vi "Modbus Message Loop.vi"(0 "Message Queues in":T1, 1 "PLC IP address":string="10.2.0.11", 3 "error in (no error)":errorcluster) -> (10 "error out":errorcluster)   [LabVIEW 2020, in "Modbus.lvlib"]
uses:
  Modbus.lvlib
  support/Message Queue/All Message Queues.ctl
  support/Message Queue/Message Cluster.ctl
  <vilib>/NI/Modbus Library/API/Master/Modbus Master.lvclass
  support/Message Queue/Enqueue Message (Single).vi
  <vilib>/NI/Modbus Library/API/Wrapper/Create TCP Master.vi
  support/Message Queue/Message Queue.lvlib
  <vilib>/NI/Modbus Library/API/Wrapper/API Main.lvlib
panel:
  out "appended array":string[](array[string])
  out "TimeoutRequestGetDataLDO":u16[](array[numeric])
  out "LDO Number":u32
  out "LDO Output":bool[](array[boolean])
  out "FV Number":u32
  out "Loop Count":i32
  out "FV Output":bool[](array[boolean])
  out "TimeoutRequestGetDataFVIR":i32[](array[numeric])
  out "Input Registers":u16[](array[numeric])
  # "Anybus: 192.168.0.50\nPLC: 192.168.0.20\n\nThis is available in the front HMI, e. IP and port. Useful for debugging and IP config change"
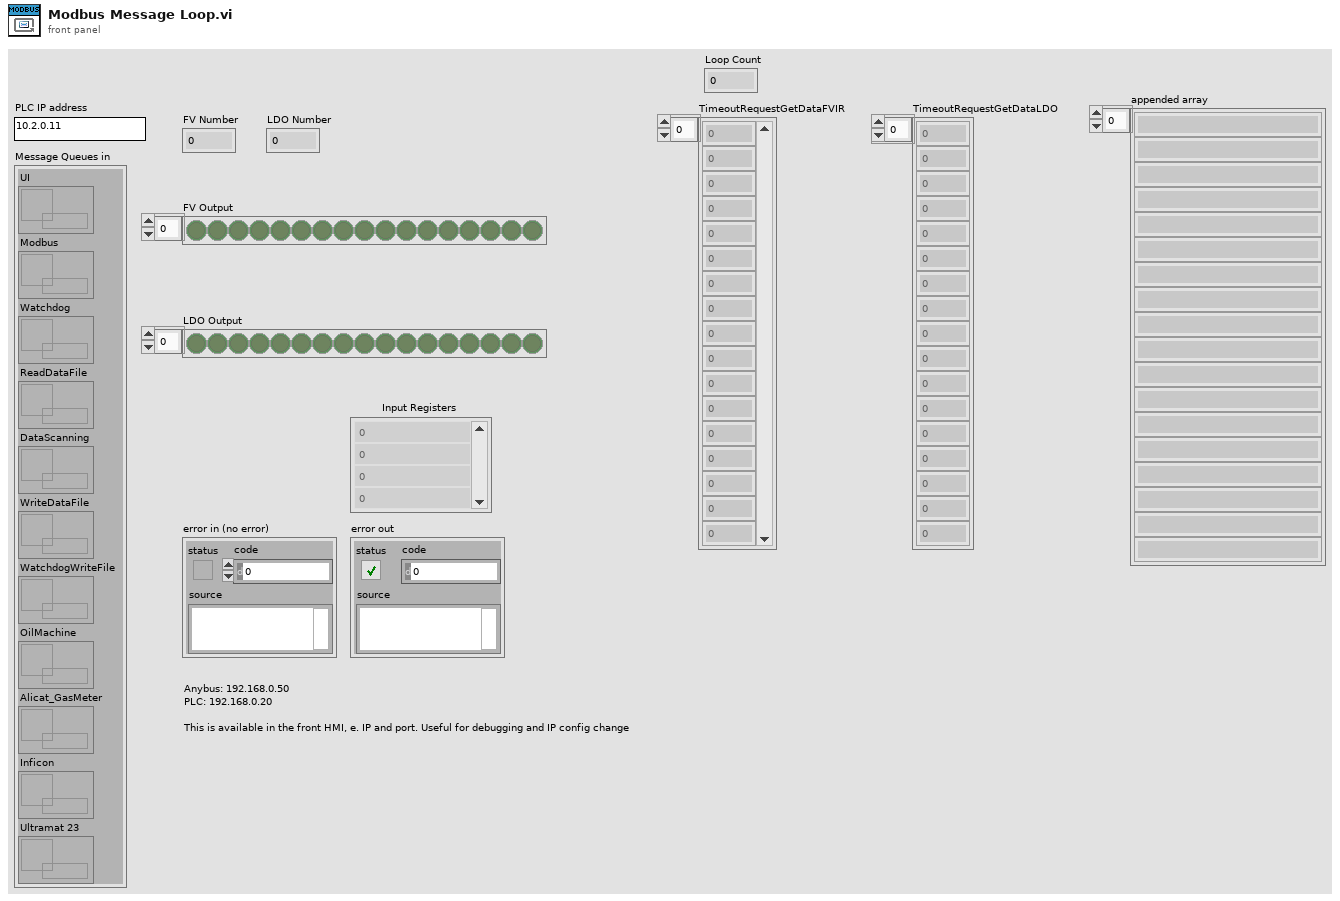
[diagram p1: front panel]
types:
  T1 = typedef "Message Queue.lvlib/All Message Queues.ctl" = cluster{"UI":refnum<queue>, "Modbus":refnum<queue>, "Watchdog":refnum<queue>, "ReadDataFile":refnum<queue>, "DataScanning":refnum<queue>, "WriteDataFile":refnum<queue>, "WatchdogWriteFile":refnum<queue>, "OilMachine":refnum<queue>, "Alicat_GasMeter":refnum<queue>, "Inficon":refnum<queue>, "Ultramat 23":refnum<queue>}
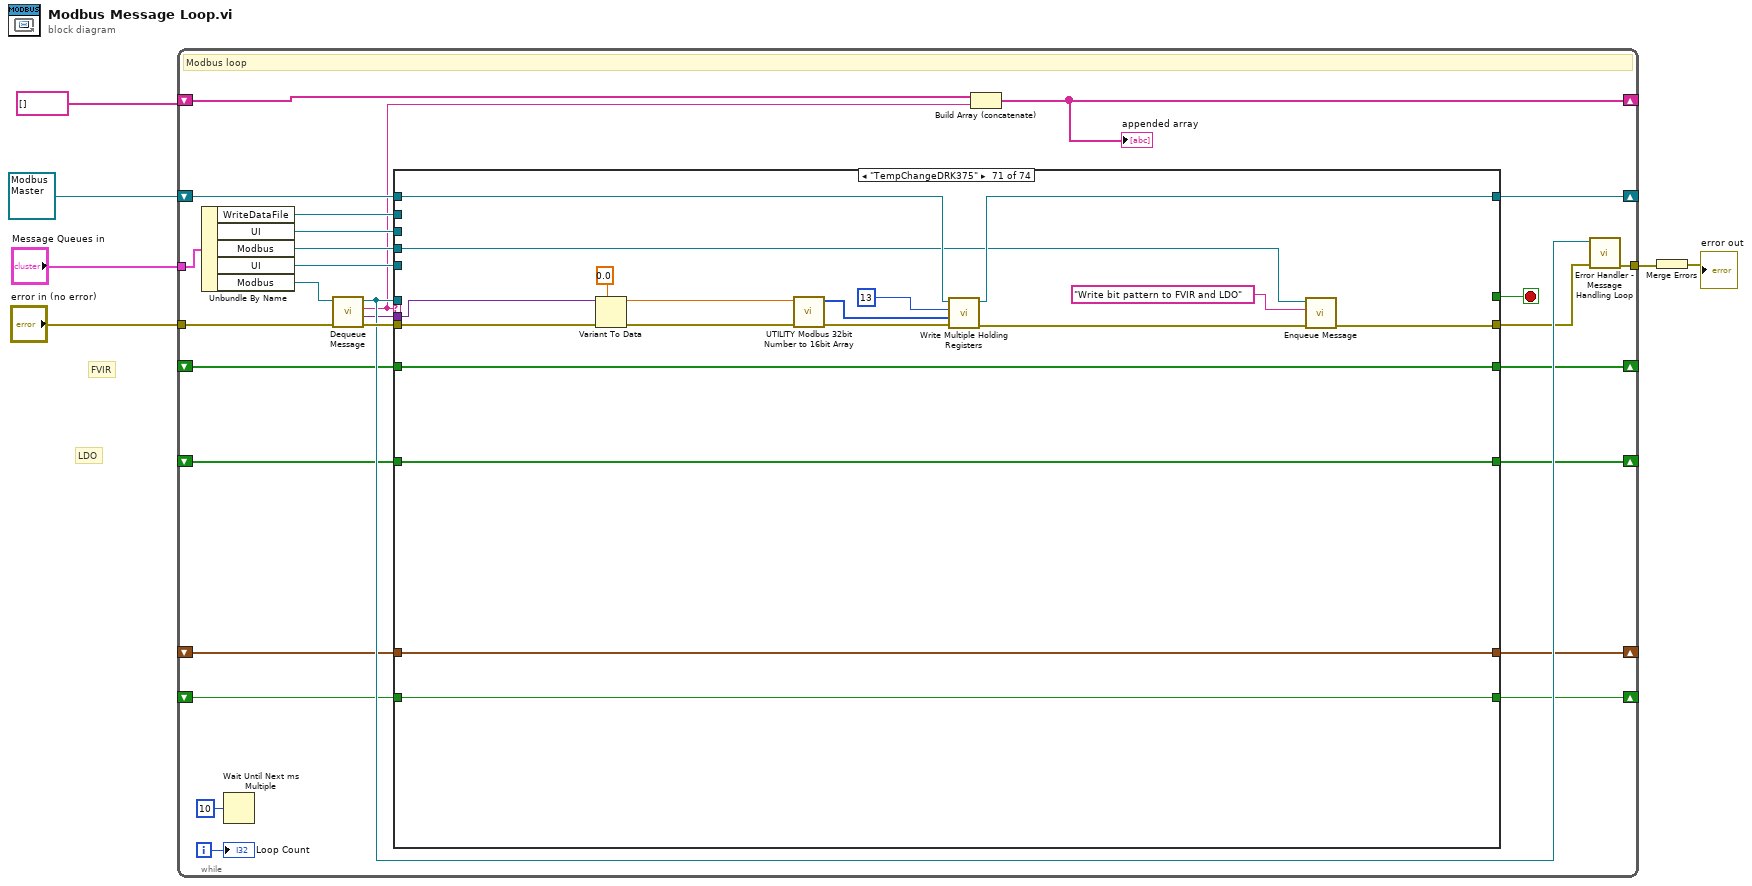
[diagram p0: block diagram]
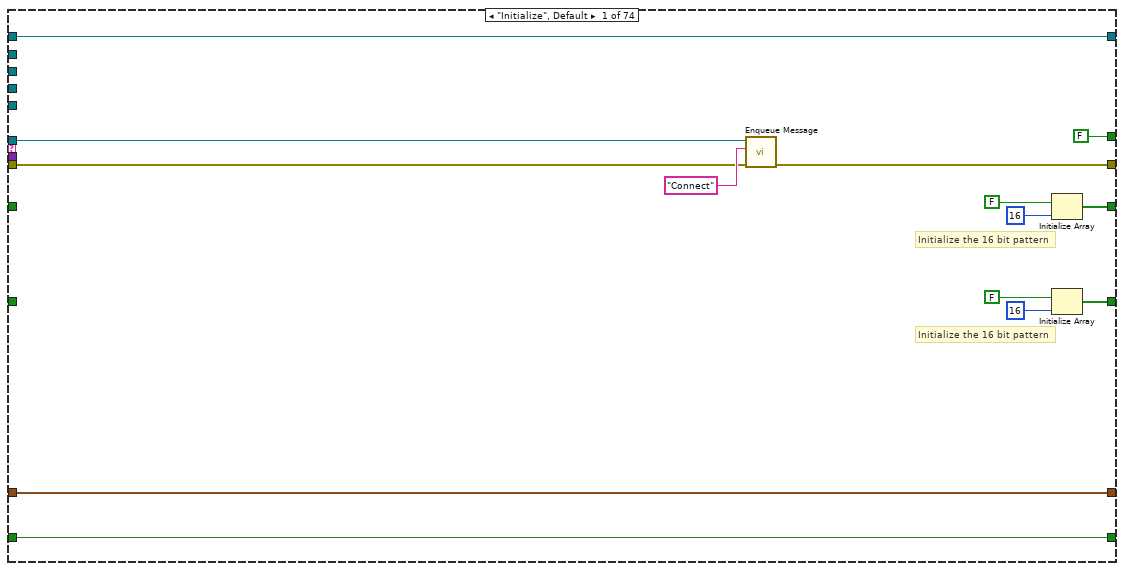
[diagram p2: hidden frame]
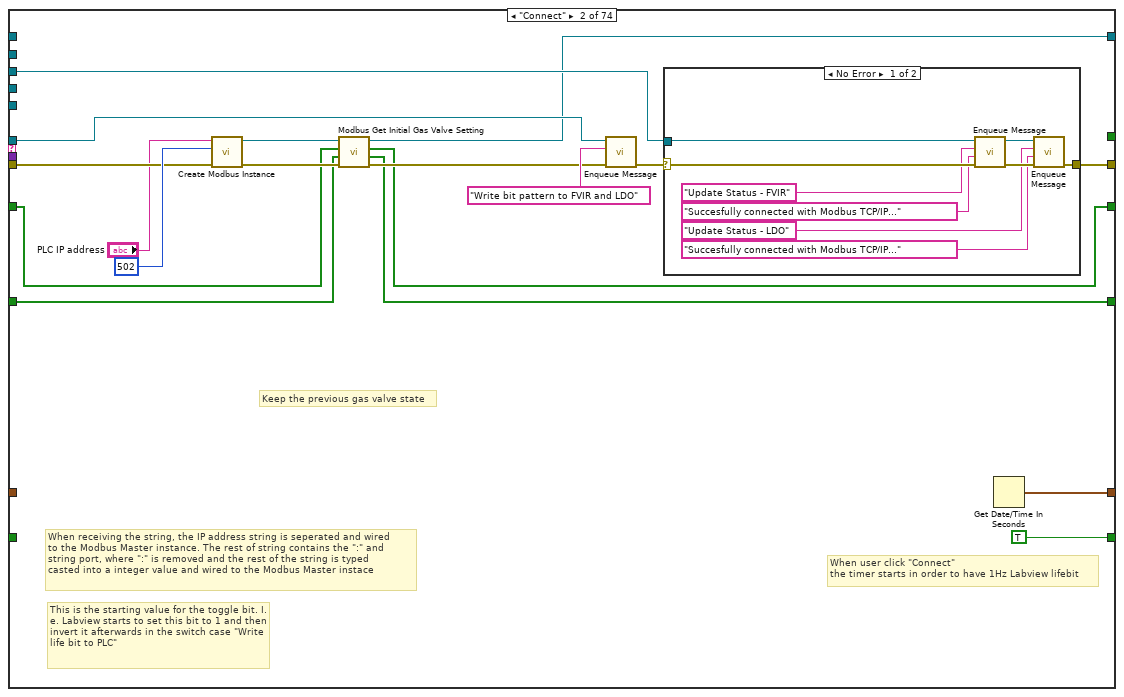
[diagram p3: hidden frame]
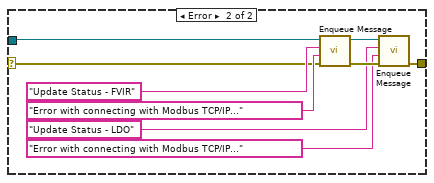
[diagram p4: hidden frame]
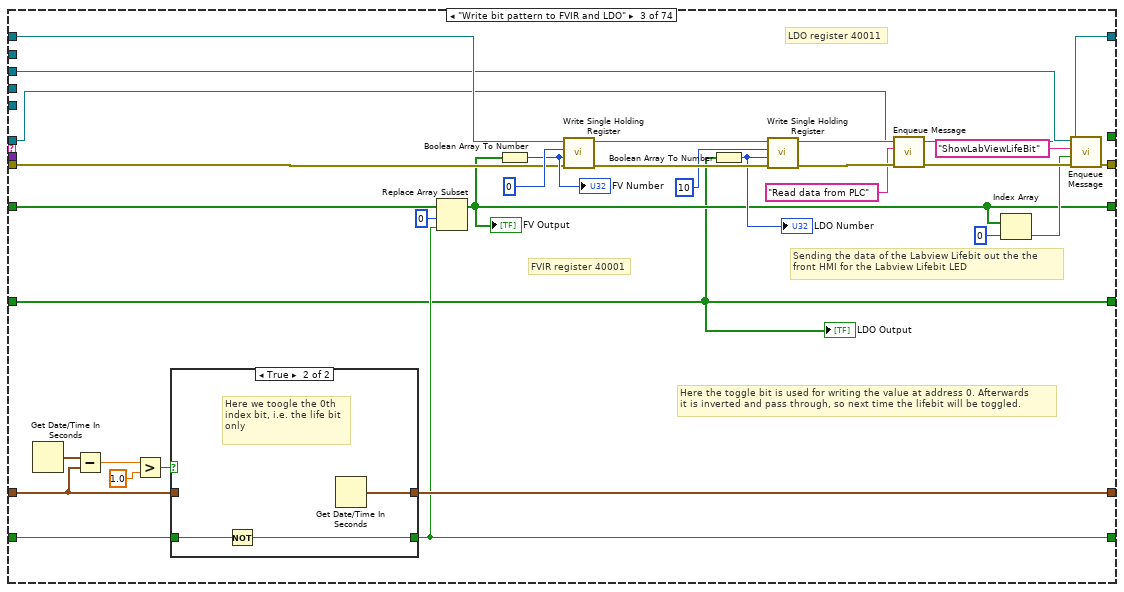
[diagram p5: hidden frame]
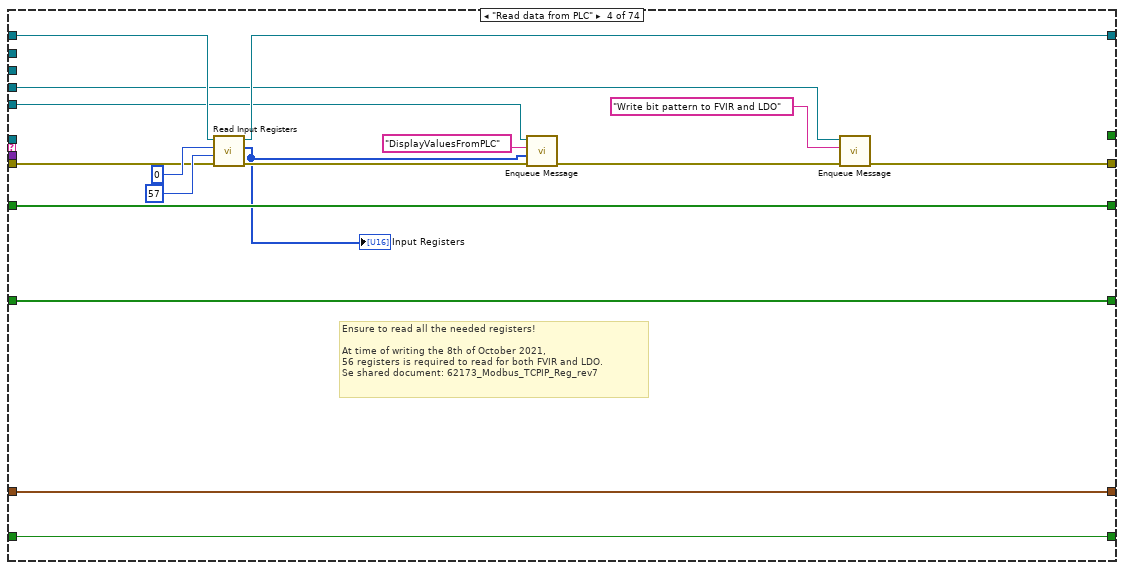
[diagram p7: hidden frame]
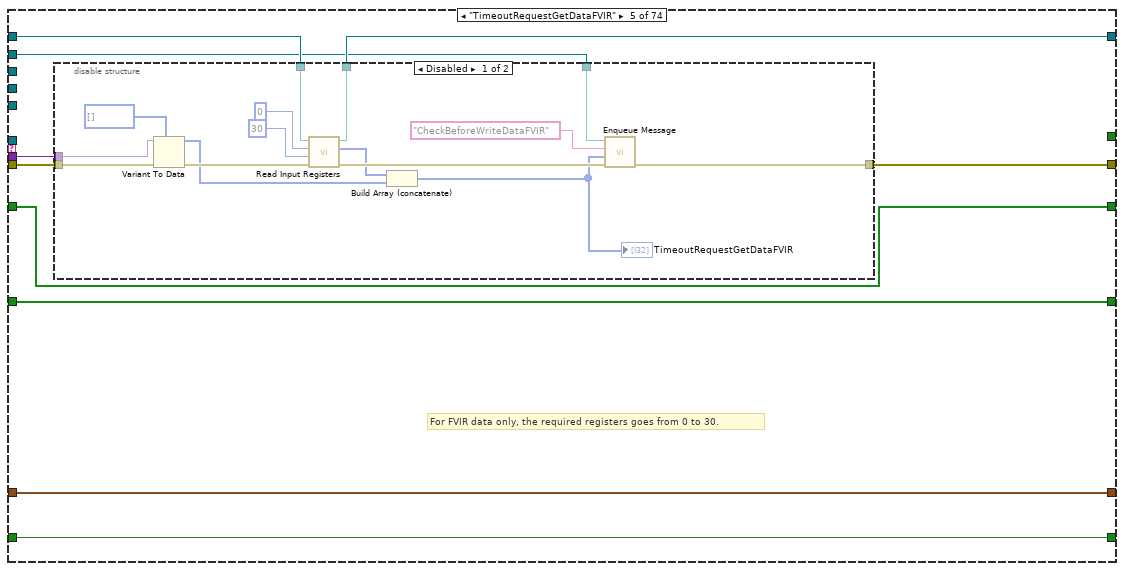
[diagram p8: hidden frame]
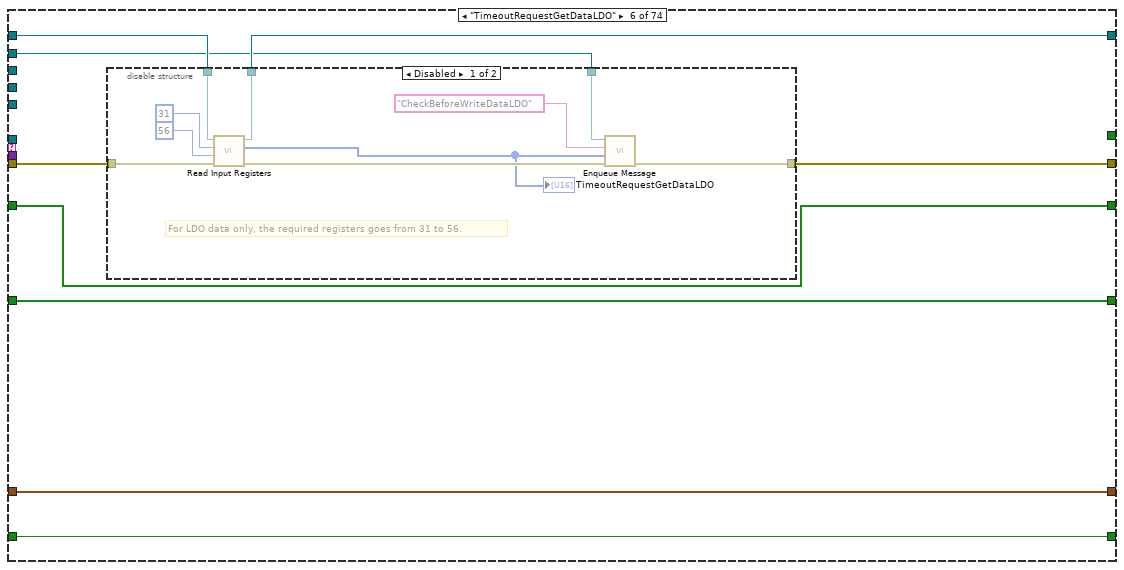
[diagram p10: hidden frame]
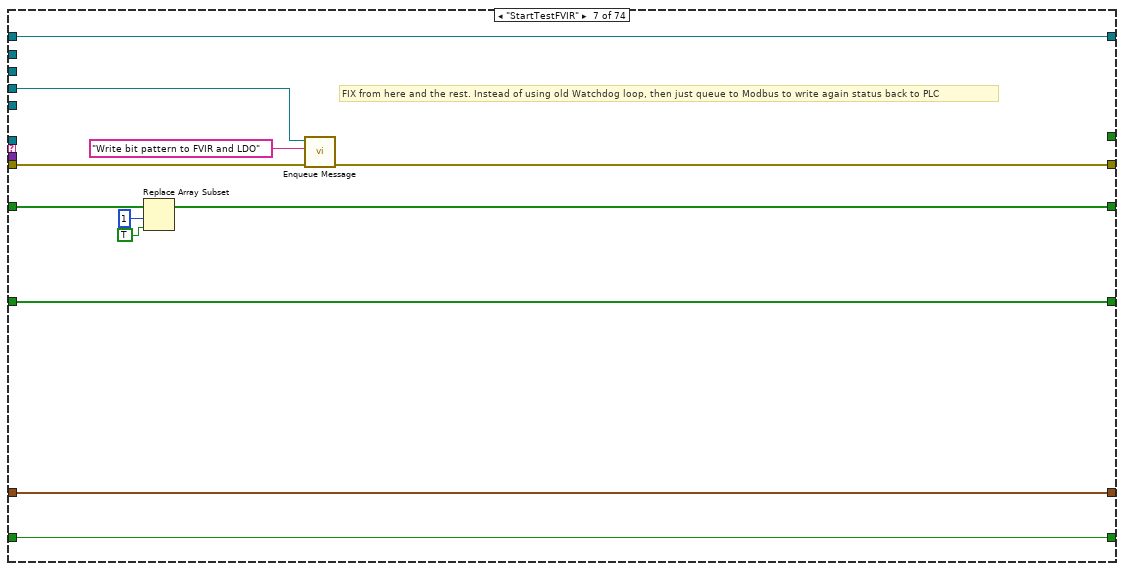
[diagram p12: hidden frame]
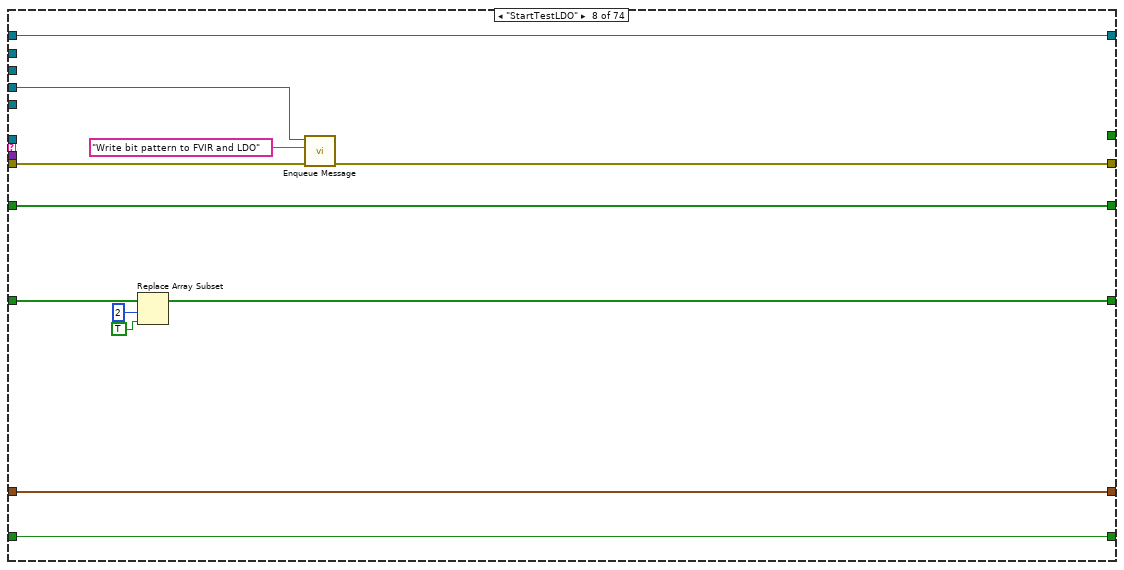
[diagram p13: hidden frame]
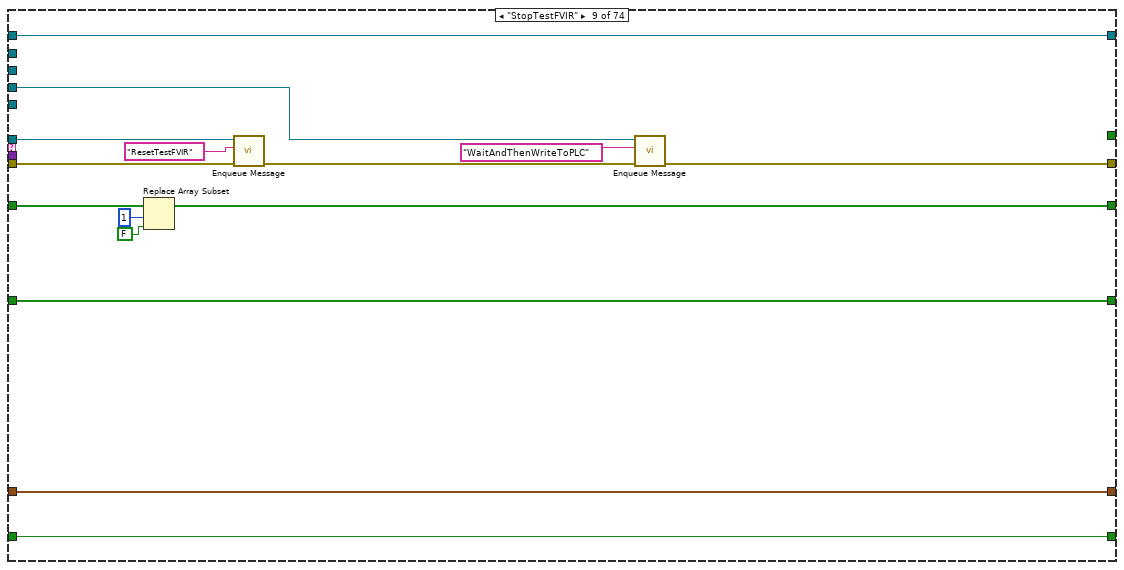
[diagram p14: hidden frame]
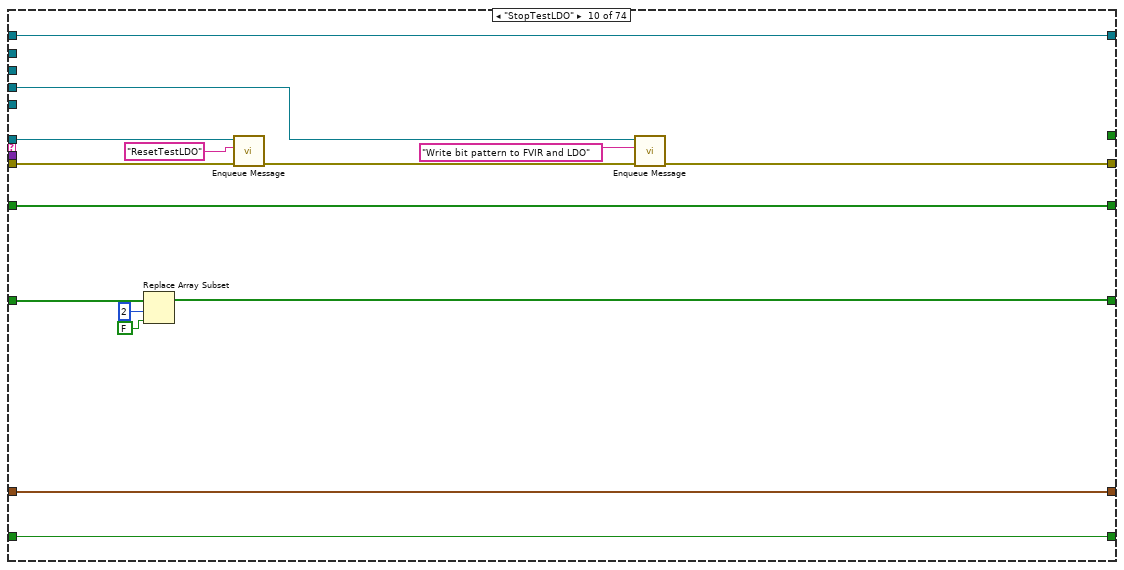
[diagram p15: hidden frame]
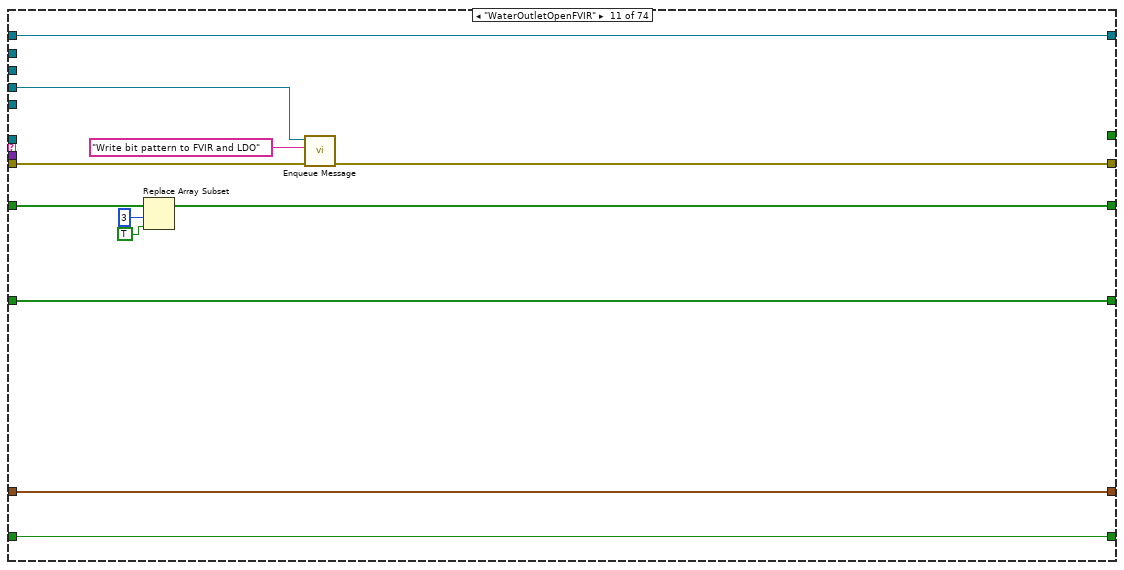
[diagram p16: hidden frame]
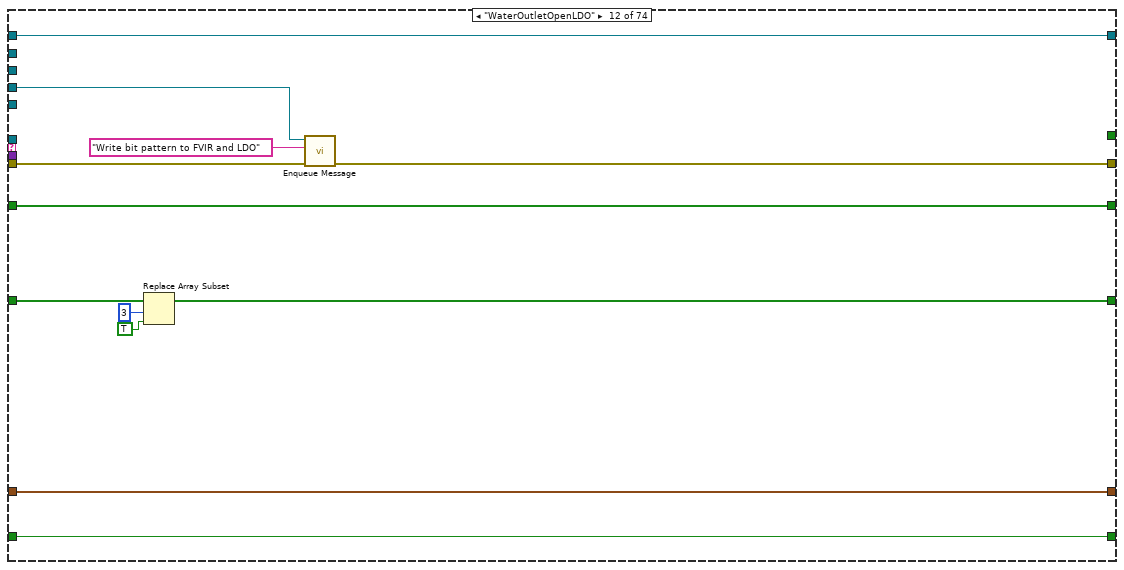
[diagram p17: hidden frame]
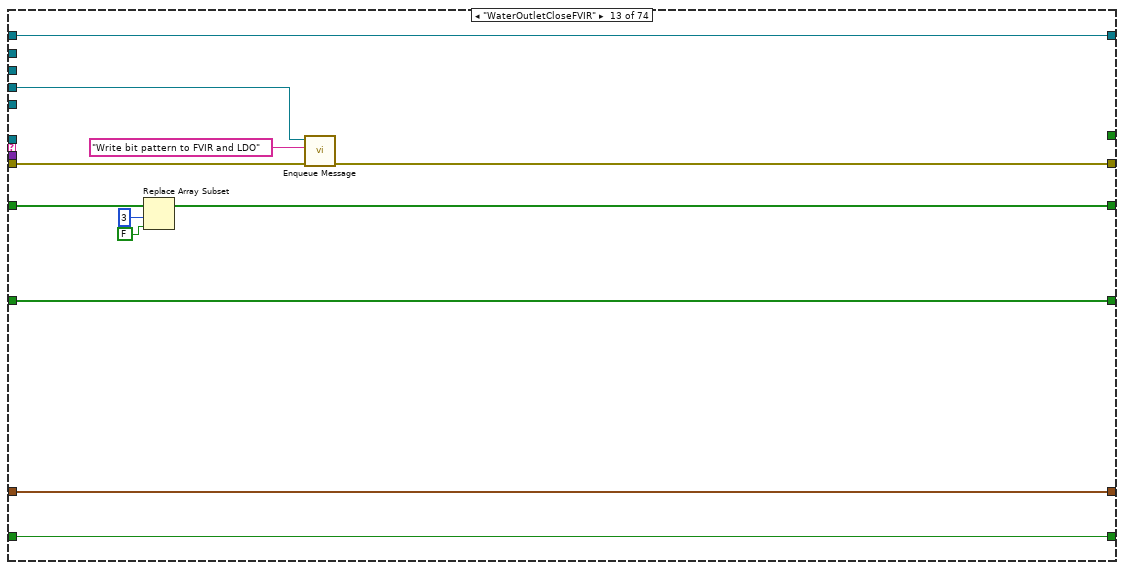
[diagram p18: hidden frame]
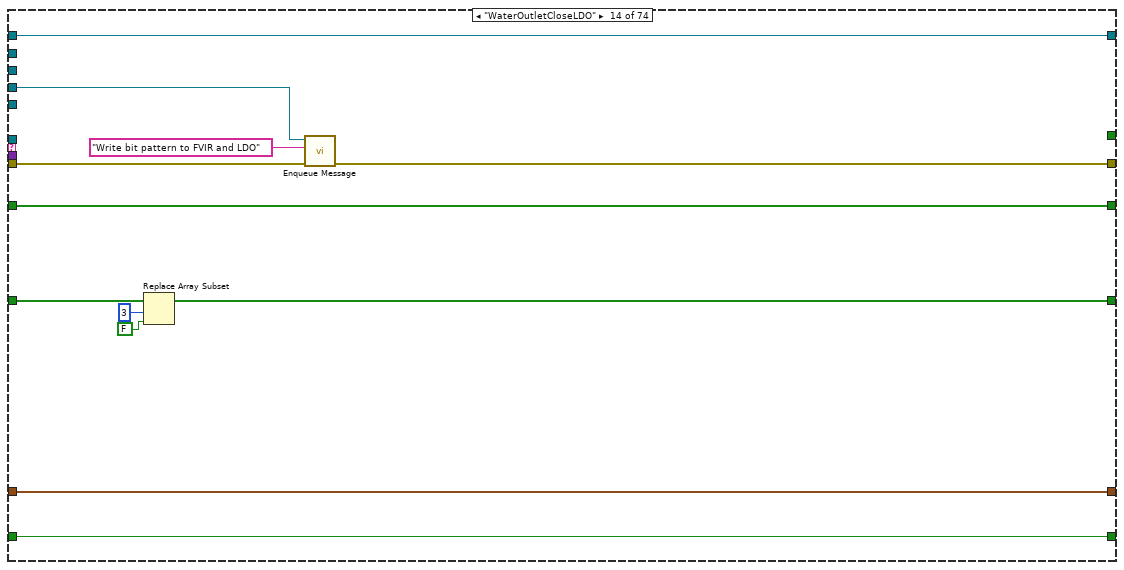
[diagram p19: hidden frame]
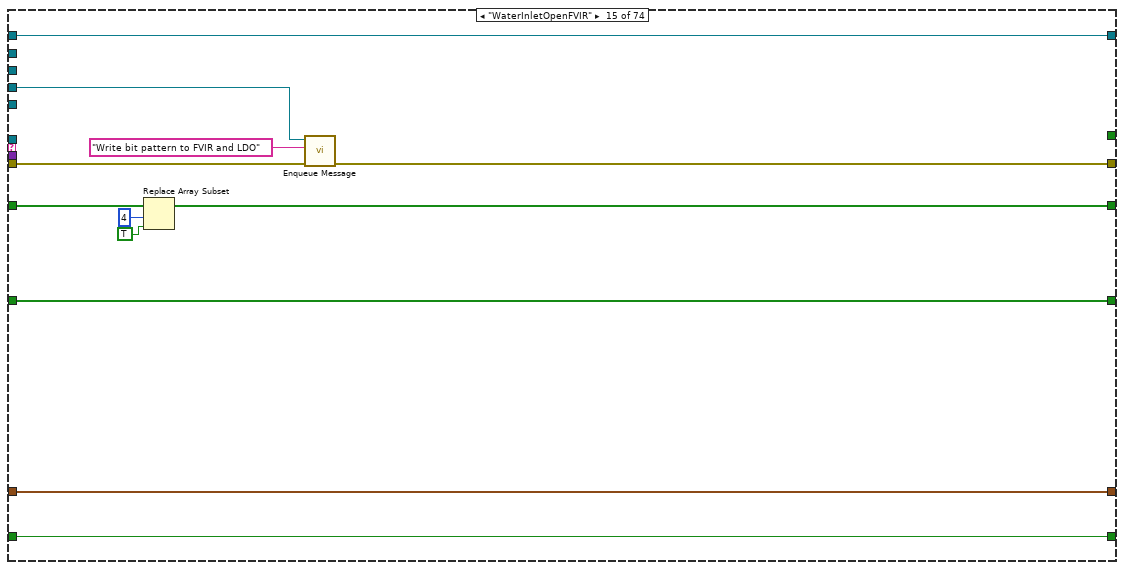
[diagram p20: hidden frame]
diagram:
  # "LDO"
  # "FVIR"
  n1 = while {
    tunnel: "Message Queues in" -> [w32]
    tunnel: [w31] -> w3
    tunnel: "error in (no error)" -> [w30]
    shift-right: [w28] -> _
    shift-left: refnum<class "Modbus Master.lvclass"> refnum ("Modbus Master") -> [w29]
    shift-right: [w22] -> _
    shift-left: _ -> [w21]
    shift-right: [w18] -> _
    shift-left: _ -> [w17]
    shift-right: [w15] -> _
    shift-left: _ -> [w14]
    shift-right: [w13] -> _
    shift-left: _ -> [w12]
    shift-right: [w7] -> _
    shift-left: string[] [] -> [w9]
    i -> [w10]
    stop <- w33 stop-if-true
    # "Modbus loop"
    n2 = Unbundle By Name(w32) -> ("WriteDataFile"=w16:refnum<queue>, "UI"=w20:refnum<queue>, "Modbus"=w26:refnum<queue>, "UI"=w24:refnum<queue>, "Modbus"=w25:refnum<queue>)
    n3 = Wait Until Next ms Multiple(millisecond multiple=u32 10) -> ()  [unwired: 1 out]
    n4 = call "Dequeue Message.vi"("error in (no error)"=w30, "Message Queue"=w25) -> ("error out"=w34:errorcluster, "Message Data"=w23:variant, "Message"=w8:string, "dup Message Queue"=w27:refnum<queue>)  [unwired: 6 in]
    n5 = case shown="\"TempChangeDRK375\"" w8 {
      tunnel: w27 -> [w35 w62 w98 _ _ _ _ _ w214 w231 _ _ _ _ _ _ _ _ _ _ _ _ _ _ _ _ _ _ _ _ _ _ _ _ _ _ _ _ _ _ _ _ _ _ _ _ _ _ _ _ _ _ _ _ _ _ _ _ _ _ _ _ _ _ _ _ _ _ w1001 _ _ _ _ _]
      tunnel: w34 -> [w37 w58 w99 w128 w140 w169 w193 w204 w213 w230 w246 w258 w270 w282 w294 w306 w318 w330 w342 w354 w366 w378 w390 w402 w414 w426 w438 w450 w462 w474 w482 w492 w510 w522 w534 w546 w558 w570 w582 w594 w601 w613 w625 w637 w649 w661 w682 w692 w708 w718 w734 w744 w760 w770 w787 w800 w813 w826 w839 w852 w857 w878 w891 w904 _ _ w952 w963 w991 w1032 w1050 w1068 w1081 w1099]
      tunnel: [w36 w65 w110 w123 w142 w167 w195 w207 w216 w233 w249 w261 w273 w285 w297 w309 w321 w333 w345 w357 w369 w381 w393 w405 w417 w429 w441 w453 w465 w477 w479 w491 w513 w525 w537 w549 w561 w573 w585 w597 w600 w612 w624 w636 w648 w660 w676 w695 w702 w721 w728 w747 w754 w773 w779 w792 w805 w818 w831 w844 w858 w870 w883 w896 w915 w938 w948 w956 w984 w1021 w1038 w1056 w1075 w1093] -> w19
      tunnel: [FALSE _ _ _ _ _ _ _ _ _ _ _ _ _ _ _ _ _ _ _ _ _ _ _ _ _ _ _ _ _ _ _ _ _ _ _ _ _ _ _ _ _ _ _ _ _ _ _ _ _ _ _ _ _ _ _ _ _ _ _ _ _ _ _ _ _ _ _ TRUE _ _ _ _ _] -> w33
      tunnel: w29 -> [w48 _ w114 w135 w146 w172 w194 w205 w222 w237 w247 w259 w271 w283 w295 w307 w319 w331 w343 w355 w367 w379 w391 w403 w415 w427 w439 w451 w463 w475 w487 w499 w511 w523 w535 w547 w559 w571 w583 w595 w599 w611 w623 w635 w647 w659 w683 w693 w709 w719 w735 w745 w761 w771 w785 w798 w811 w824 w837 w850 w864 w876 w889 w902 w912 w936 w950 w962 w987 w1025 w1043 w1061 w1079 w1097]
      tunnel: [w48 w53 w102 w133 w145 w171 w194 w205 w222 w237 w247 w259 w271 w283 w295 w307 w319 w331 w343 w355 w367 w379 w391 w403 w415 w427 w439 w451 w463 w475 w487 w499 w511 w523 w535 w547 w559 w571 w583 w595 w599 w611 w623 w635 w647 w659 w683 w693 w709 w719 w735 w745 w761 w771 w786 w799 w812 w825 w838 w851 w865 w877 w890 w903 w911 w935 w951 w962 w987 w1024 w1042 w1060 w1078 w1096] -> w28
      tunnel: w26 -> [_ _ _ w122 _ _ w196 w208 w217 w234 w250 w262 w274 w286 w298 w310 w322 w334 w346 w358 w370 w382 w394 w406 w418 w430 w442 w454 w466 w478 w483 w493 w514 w526 w538 w550 w562 w574 w586 w598 w602 w614 w626 w638 w650 w662 w675 w696 w701 w722 w727 w748 w753 w774 w782 w795 w808 w821 w834 w847 w861 w873 w886 w899 w919 w942 _ w960 w990 w1020 w1040 w1058 w1074 w1092]
      tunnel: w24 -> [_ _ _ w131 _ _ _ _ _ _ _ _ _ _ _ _ _ _ _ _ _ _ _ _ _ _ _ _ _ _ _ _ _ _ _ _ _ _ _ _ _ _ _ _ _ _ _ _ _ _ _ _ _ _ _ _ _ _ _ _ _ _ _ _ _ _ _ _ w983 _ _ _ _ _]
      tunnel: w23 -> [_ _ _ _ w139 _ _ _ _ _ _ _ _ _ _ _ _ _ _ _ _ _ _ _ _ _ _ _ _ _ _ _ _ _ _ _ _ _ _ _ _ _ _ _ _ _ _ _ _ _ _ _ _ _ _ _ _ _ _ _ _ _ _ _ w917 w940 _ _ _ w1031 w1049 w1067 w1080 w1098]
      tunnel: [w44 w51 w88 w129 w144 w170 w190 w199 w219 w228 w243 w253 w267 w277 w291 w301 w315 w325 w339 w349 w363 w373 w387 w397 w411 w421 w435 w445 w459 w469 w490 w502 w505 w517 w529 w541 w553 w565 w577 w589 w610 w622 w634 w646 w658 w670 w679 w689 w705 w715 w731 w741 w757 w767 w778 w791 w804 w817 w830 w843 w856 w869 w882 w895 w908 w932 w946 w959 w996 w1037 w1055 w1073 w1091 w1109] -> w22
      tunnel: w21 -> [_ w52 w89 w129 w144 w170 w191 w199 w220 w228 w244 w253 w268 w277 w292 w301 w316 w325 w340 w349 w364 w373 w388 w397 w412 w421 w436 w445 w460 w469 w490 w502 w505 w517 w529 w541 w553 w565 w577 w589 w610 w622 w634 w646 w658 w670 w680 w690 w706 w716 w732 w742 w758 w768 w778 w791 w804 w817 w830 w843 w856 w869 w882 w895 w908 w932 w946 w959 w996 w1037 w1055 w1073 w1091 w1109]
      tunnel: w20 -> [_ w66 w108 _ _ _ _ _ _ _ _ _ _ _ _ _ _ _ _ _ _ _ _ _ _ _ _ _ _ _ _ _ _ _ _ _ _ _ _ _ _ _ _ _ _ _ _ _ _ _ _ _ _ _ _ _ _ _ _ _ _ _ _ _ _ _ _ w955 _ _ _ _ _ _]
      tunnel: [w41 w49 w85 w125 w143 w168 w188 w200 w211 w226 w241 w254 w265 w278 w289 w302 w313 w326 w337 w350 w361 w374 w385 w398 w409 w422 w433 w446 w457 w470 w480 w494 w506 w518 w530 w542 w554 w566 w578 w590 w604 w616 w628 w640 w652 w664 w673 w687 w699 w713 w725 w739 w751 w765 w777 w790 w803 w816 w829 w842 w855 w868 w881 w894 w907 w931 w945 w958 w995 w1036 w1054 w1072 w1090 w1108] -> w18
      tunnel: w17 -> [_ w50 w85 w125 w143 w168 w188 w201 w211 w227 w241 w255 w265 w279 w289 w303 w313 w327 w337 w351 w361 w375 w385 w399 w409 w423 w433 w447 w457 w471 w481 w495 w507 w519 w531 w543 w555 w567 w579 w591 w605 w617 w629 w641 w653 w665 w673 w687 w699 w713 w725 w739 w751 w765 w777 w790 w803 w816 w829 w842 w855 w868 w881 w894 w907 w931 w945 w958 w995 w1036 w1054 w1072 w1090 w1108]
      tunnel: w16 -> [_ _ _ _ w141 w166 _ _ _ _ _ _ _ _ _ _ _ _ _ _ _ _ _ _ _ _ _ _ _ _ _ _ _ _ _ _ _ _ _ _ _ _ _ _ _ _ _ _ _ _ _ _ _ _ _ _ _ _ _ _ _ _ _ _ _ _ _ _ _ _ _ _ _ _]
      tunnel: [w40 w61 w92 w121 w138 w165 w186 w198 w210 w225 w240 w252 w264 w276 w288 w300 w312 w324 w336 w348 w360 w372 w384 w396 w408 w420 w432 w444 w456 w468 w489 w501 w504 w516 w528 w540 w552 w564 w576 w588 w609 w621 w633 w645 w657 w669 w672 w686 w698 w712 w724 w738 w750 w764 w776 w789 w802 w815 w828 w841 w854 w867 w880 w893 w906 w930 w944 w954 w994 w1035 w1053 w1071 w1089 w1107] -> w15
      tunnel: w14 -> [w40 _ w91 w121 w138 w165 w186 w198 w210 w225 w240 w252 w264 w276 w288 w300 w312 w324 w336 w348 w360 w372 w384 w396 w408 w420 w432 w444 w456 w468 w489 w501 w504 w516 w528 w540 w552 w564 w576 w588 w609 w621 w633 w645 w657 w669 w672 w686 w698 w712 w724 w738 w750 w764 w776 w789 w802 w815 w828 w841 w854 w867 w880 w893 w906 w930 w944 w954 w994 w1035 w1053 w1071 w1089 w1107]
      tunnel: [w39 TRUE w86 w120 w137 w164 w185 w197 w209 w224 w239 w251 w263 w275 w287 w299 w311 w323 w335 w347 w359 w371 w383 w395 w407 w419 w431 w443 w455 w467 w488 w500 w503 w515 w527 w539 w551 w563 w575 w587 w608 w620 w632 w644 w656 w668 w671 w685 w697 w711 w723 w737 w749 w763 w775 w788 w801 w814 w827 w840 w853 w866 w879 w892 w905 w929 w943 w953 w993 w1034 w1052 w1070 w1088 w1106] -> w13
      tunnel: w12 -> [w39 _ w90 w120 w137 w164 w185 w197 w209 w224 w239 w251 w263 w275 w287 w299 w311 w323 w335 w347 w359 w371 w383 w395 w407 w419 w431 w443 w455 w467 w488 w500 w503 w515 w527 w539 w551 w563 w575 w587 w608 w620 w632 w644 w656 w668 w671 w685 w697 w711 w723 w737 w749 w763 w775 w788 w801 w814 w827 w840 w853 w866 w879 w892 w905 w929 w943 w953 w993 w1034 w1052 w1070 w1088 w1106]
      frame "Initialize", Default {
        # "Initialize the 16 bit pattern"
        # "Initialize the 16 bit pattern"
        n6 = call-poly "Enqueue Message.vi"("error in (no error)"=w37, "Message"="Connect", "Message Queue"=w35) -> ("error out"=w36:errorcluster)  [unwired: 7 in, 1 out]
        n7 = Initialize Array(FALSE, 16 ("dimension size")) -> (w44:bool[])
        n8 = Initialize Array(FALSE, 16 ("dimension size")) -> (w41:bool[])
      }
      frame "Connect" {
        # "Keep the previous gas valve state"
        # "When user click \"Connect\"\nthe timer starts in order to have 1Hz Labview lifebit"
        # "When receiving the string, the IP address string is seperated and wired\nto the Modbus Master instance. The rest of string contains the \":\" and\nstring port, where \":\" is removed and the rest of the string is typed \ncasted into a integer value and wired to the Modbus Master instace"
        # "This is the starting value for the toggle bit. I.e. Labview starts to set this bit to 1 and then invert it afterwards in the switch case \"Write life bit to PLC\""
        n9 = call-poly <vilib>:"Create Modbus Instance.vi"("error in"=w58, "port (502)"=u16 502 ("Port"), "address"="PLC IP address") -> ("error out"=w56:errorcluster, "TCP master instance"=w54:refnum<class "Modbus Master.lvclass">)  [unwired: 7 in]
        n10 = call "Modbus Get Initial Gas Valve Setting.vi"("error in (no error)"=w56, "LDO Input"=w50, "FVIR Input"=w52, "Modbus Master in"=w54) -> ("error out"=w55:errorcluster, "LDO Output"=w49:bool[], "FVIR Output"=w51:bool[], "Modbus Master out"=w53:refnum<class "Modbus Master.lvclass">)  [unwired: 4 in]
        n11 = call-poly "Enqueue Message.vi"("error in (no error)"=w55, "Message"="Write bit pattern to FVIR and LDO", "Message Queue"=w62) -> ("error out"=w63:errorcluster)  [unwired: 7 in, 1 out]
        n12 = case shown="No Error" w63 {
          selector: w63 -> [w75 w78]
          tunnel: w66 -> [w67 w76]
          tunnel: [w73 w77] -> w65
          frame No Error {
            n13 = call-poly "Enqueue Message.vi"("error in (no error)"=w75, "Message Data"="Succesfully connected with Modbus TCP/IP..." ("Acquiring and Logging..."), "Message"="Update Status - FVIR", "Message Queue"=w67) -> ("error out"=w74:errorcluster, "dup Message Queue"=w72:refnum<queue>)  [unwired: 6 in]
            n14 = call-poly "Enqueue Message.vi"("error in (no error)"=w74, "Message Data"="Succesfully connected with Modbus TCP/IP..." ("Acquiring and Logging..."), "Message"="Update Status - LDO", "Message Queue"=w72) -> ("error out"=w73:errorcluster)  [unwired: 6 in, 1 out]
          }
          frame Error {
            n15 = call-poly "Enqueue Message.vi"("error in (no error)"=w78, "Message Data"="Error with connecting with Modbus TCP/IP..." ("Acquiring and Logging..."), "Message"="Update Status - FVIR", "Message Queue"=w76) -> ("error out"=w84:errorcluster, "dup Message Queue"=w83:refnum<queue>)  [unwired: 6 in]
            n16 = call-poly "Enqueue Message.vi"("error in (no error)"=w84, "Message Data"="Error with connecting with Modbus TCP/IP..." ("Acquiring and Logging..."), "Message"="Update Status - LDO", "Message Queue"=w83) -> ("error out"=w77:errorcluster)  [unwired: 6 in, 1 out]
          }
        }
        n17 = Get Date/Time In Seconds() -> (seconds since 1Jan1904=w61:timestamp)
      }
      frame "Write bit pattern to FVIR and LDO" {
        # "LDO register 40011"
        # "FVIR register 40001"
        # "Sending the data of the Labview Lifebit out the the \nfront HMI for the Labview Lifebit LED"
        # "Here the toggle bit is used for writing the value at address 0. Afterwards\nit is inverted and pass through, so next time the lifebit will be toggled."
        n18 = Get Date/Time In Seconds() -> (seconds since 1Jan1904=w96:timestamp)
        n19 = Subtract(x=w96, y=w91) -> (x-y=w95:dbl)
        n20 = Greater?(x=w95, y=1.0) -> (0:w93:bool)
        n21 = case shown="True" w93 {
          tunnel: w91 -> [w115 _]
          tunnel: [w115 w119] -> w92
          tunnel: w90 -> [w116 w118]
          tunnel: [w116 w117] -> w86
          frame False {
          }
          frame True {
            # "Here we toogle the 0th index bit, i.e. the life bit only"
            n22 = Not(x=w118) -> (.not. x?=w117:bool)
            n23 = Get Date/Time In Seconds() -> (seconds since 1Jan1904=w119:timestamp)
          }
        }
        n24 = Replace Array Subset(array=w89, new element=w86, index=0) -> (w88:bool[])
        "FV Output" <- w88
        n25 = Boolean Array To Number(Boolean array=w88) -> (number=w112:u32)
        "FV Number" <- w112
        n26 = call-dynamic "Write Single Holding Register.vi"("error in"=w99, "register to write"=w112, "address"=u16 0 ("starting address"), "Modbus master in"=w114) -> ("error out"=w104:errorcluster, "Modbus master out"=w105:refnum<class "Modbus Master.lvclass">)  [unwired: 6 in]
        n27 = Boolean Array To Number(Boolean array=w85) -> (number=w100:u32)
        "LDO Number" <- w100
        n28 = call-dynamic "Write Single Holding Register.vi"("error in"=w104, "register to write"=w100, "address"=u16 10, "Modbus master in"=w105) -> ("error out"=w103:errorcluster, "Modbus master out"=w102:refnum<class "Modbus Master.lvclass">)  [unwired: 6 in]
        n29 = call-poly "Enqueue Message.vi"("error in (no error)"=w103, "Message"="Read data from PLC", "Message Queue"=w98) -> ("error out"=w111:errorcluster)  [unwired: 7 in, 1 out]
        n30 = Index Array(array=w88, index=0) -> (element=w106:bool)
        n31 = call-poly "Enqueue Message.vi"("error in (no error)"=w111, "Message Data"=w106, "Message"="ShowLabViewLifeBit", "Message Queue"=w108) -> ("error out"=w110:errorcluster)  [unwired: 6 in, 1 out]
        "LDO Output" <- w85
      }
      frame "Read data from PLC" {
        # "Ensure to read all the needed registers! \n\nAt time of writing the 8th of October 2021, \n56 registers is required to read for both FVIR and LDO. \nSe shared document: 62173_Modbus_TCPIP_Reg_rev7"
        n32 = call-dynamic "Read Input Registers.vi"("error in"=w128, "number of inputs"=u16 57, "starting address"=u16 0, "Modbus master in"=w135) -> ("error out"=w127:errorcluster, "register values"=w124:u16[], "Modbus master out"=w133:refnum<class "Modbus Master.lvclass">)  [unwired: 5 in]
        "Input Registers" <- w124
        n33 = call-poly "Enqueue Message.vi"("error in (no error)"=w127, "Message Data"=w124, "Message"="DisplayValuesFromPLC", "Message Queue"=w131) -> ("error out"=w126:errorcluster)  [unwired: 6 in, 1 out]
        n34 = call-poly "Enqueue Message.vi"("error in (no error)"=w126, "Message"="Write bit pattern to FVIR and LDO", "Message Queue"=w122) -> ("error out"=w123:errorcluster)  [unwired: 7 in, 1 out]
      }
      frame "TimeoutRequestGetDataFVIR" {
        # "For FVIR data only, the required registers goes from 0 to 30."
        n35 = disable-structure shown="Disabled" {
          disable-tunnel: w146 -> [w160 w163]
          disable-tunnel: [w158 w163] -> w145
          disable-tunnel: [w156 w162] -> w142
          disable-tunnel: w141 -> [w155 _]
          disable-tunnel: w140 -> [w153 w162]
          disable-tunnel: w139 -> [w150 _]
          frame Disabled {
            n36 = Variant To Data(error in=w153, type=i32[] [], Variant=w150) -> (data=w148:i32[], error out=w152:errorcluster)
            n37 = call-dynamic "Read Input Registers.vi"("error in"=w152, "number of inputs"=u16 30, "starting address"=u16 0, "Modbus master in"=w160) -> ("error out"=w157:errorcluster, "register values"=w149:u16[], "Modbus master out"=w158:refnum<class "Modbus Master.lvclass">)  [unwired: 5 in]
            n38 = Build Array (concatenate)(w149, w148) -> (w147:i32[])
            "TimeoutRequestGetDataFVIR" <- w147
            n39 = call-poly "Enqueue Message.vi"("error in (no error)"=w157, "Message Data"=w147, "Message"="CheckBeforeWriteDataFVIR", "Message Queue"=w155) -> ("error out"=w156:errorcluster)  [unwired: 6 in, 1 out]
          }
          frame Enabled {
          }
        }
      }
      frame "TimeoutRequestGetDataLDO" {
        n40 = disable-structure shown="Disabled" {
          disable-tunnel: w172 -> [w181 w183]
          disable-tunnel: [w179 w183] -> w171
          disable-tunnel: w169 -> [w178 w184]
          disable-tunnel: [w176 w184] -> w167
          disable-tunnel: w166 -> [w175 _]
          frame Disabled {
            # "For LDO data only, the required registers goes from 31 to 56."
            n41 = call-dynamic "Read Input Registers.vi"("error in"=w178, "number of inputs"=u16 56, "starting address"=u16 31, "Modbus master in"=w181) -> ("error out"=w177:errorcluster, "register values"=w174:u16[], "Modbus master out"=w179:refnum<class "Modbus Master.lvclass">)  [unwired: 5 in]
            "TimeoutRequestGetDataLDO" <- w174
            n42 = call-poly "Enqueue Message.vi"("error in (no error)"=w177, "Message Data"=w174, "Message"="CheckBeforeWriteDataLDO", "Message Queue"=w175) -> ("error out"=w176:errorcluster)  [unwired: 6 in, 1 out]
          }
          frame Enabled {
          }
        }
      }
      frame "StartTestFVIR" {
        # "FIX from here and the rest. Instead of using old Watchdog loop, then just queue to Modbus to write again status back to PLC"
        n43 = Replace Array Subset(array=w191, new element=TRUE ("new element/subarray"), index=1) -> (w190:bool[])
        n44 = call-poly "Enqueue Message.vi"("error in (no error)"=w193, "Message"="Write bit pattern to FVIR and LDO", "Message Queue"=w196) -> ("error out"=w195:errorcluster)  [unwired: 7 in, 1 out]
      }
      frame "StartTestLDO" {
        n45 = Replace Array Subset(array=w201, new element=TRUE ("new element/subarray"), index=2) -> (w200:bool[])
        n46 = call-poly "Enqueue Message.vi"("error in (no error)"=w204, "Message"="Write bit pattern to FVIR and LDO", "Message Queue"=w208) -> ("error out"=w207:errorcluster)  [unwired: 7 in, 1 out]
      }
      frame "StopTestFVIR" {
        n47 = Replace Array Subset(array=w220, new element=FALSE ("new element/subarray"), index=1) -> (w219:bool[])
        n48 = call-poly "Enqueue Message.vi"("error in (no error)"=w213, "Message"="ResetTestFVIR", "Message Queue"=w214) -> ("error out"=w212:errorcluster)  [unwired: 7 in, 1 out]
        n49 = call-poly "Enqueue Message.vi"("error in (no error)"=w212, "Message"="WaitAndThenWriteToPLC", "Message Queue"=w217) -> ("error out"=w216:errorcluster)  [unwired: 7 in, 1 out]
      }
      frame "StopTestLDO" {
        n50 = Replace Array Subset(array=w227, new element=FALSE ("new element/subarray"), index=2) -> (w226:bool[])
        n51 = call-poly "Enqueue Message.vi"("error in (no error)"=w230, "Message"="ResetTestLDO", "Message Queue"=w231) -> ("error out"=w229:errorcluster)  [unwired: 7 in, 1 out]
        n52 = call-poly "Enqueue Message.vi"("error in (no error)"=w229, "Message"="Write bit pattern to FVIR and LDO", "Message Queue"=w234) -> ("error out"=w233:errorcluster)  [unwired: 7 in, 1 out]
      }
      frame "WaterOutletOpenFVIR" {
        n53 = Replace Array Subset(array=w244, new element=TRUE ("new element/subarray"), index=3) -> (w243:bool[])
        n54 = call-poly "Enqueue Message.vi"("error in (no error)"=w246, "Message"="Write bit pattern to FVIR and LDO", "Message Queue"=w250) -> ("error out"=w249:errorcluster)  [unwired: 7 in, 1 out]
      }
      frame "WaterOutletOpenLDO" {
        n55 = Replace Array Subset(array=w255, new element=TRUE ("new element/subarray"), index=3) -> (w254:bool[])
        n56 = call-poly "Enqueue Message.vi"("error in (no error)"=w258, "Message"="Write bit pattern to FVIR and LDO", "Message Queue"=w262) -> ("error out"=w261:errorcluster)  [unwired: 7 in, 1 out]
      }
      frame "WaterOutletCloseFVIR" {
        n57 = Replace Array Subset(array=w268, new element=FALSE ("new element/subarray"), index=3) -> (w267:bool[])
        n58 = call-poly "Enqueue Message.vi"("error in (no error)"=w270, "Message"="Write bit pattern to FVIR and LDO", "Message Queue"=w274) -> ("error out"=w273:errorcluster)  [unwired: 7 in, 1 out]
      }
      frame "WaterOutletCloseLDO" {
        n59 = Replace Array Subset(array=w279, new element=FALSE ("new element/subarray"), index=3) -> (w278:bool[])
        n60 = call-poly "Enqueue Message.vi"("error in (no error)"=w282, "Message"="Write bit pattern to FVIR and LDO", "Message Queue"=w286) -> ("error out"=w285:errorcluster)  [unwired: 7 in, 1 out]
      }
      frame "WaterInletOpenFVIR" {
        n61 = Replace Array Subset(array=w292, new element=TRUE ("new element/subarray"), index=4) -> (w291:bool[])
        n62 = call-poly "Enqueue Message.vi"("error in (no error)"=w294, "Message"="Write bit pattern to FVIR and LDO", "Message Queue"=w298) -> ("error out"=w297:errorcluster)  [unwired: 7 in, 1 out]
      }
      frame "WaterInletOpenLDO" {
        n63 = Replace Array Subset(array=w303, new element=TRUE ("new element/subarray"), index=4) -> (w302:bool[])
        n64 = call-poly "Enqueue Message.vi"("error in (no error)"=w306, "Message"="Write bit pattern to FVIR and LDO", "Message Queue"=w310) -> ("error out"=w309:errorcluster)  [unwired: 7 in, 1 out]
      }
      frame "WaterInletCloseFVIR" {
        n65 = Replace Array Subset(array=w316, new element=FALSE ("new element/subarray"), index=4) -> (w315:bool[])
        n66 = call-poly "Enqueue Message.vi"("error in (no error)"=w318, "Message"="Write bit pattern to FVIR and LDO", "Message Queue"=w322) -> ("error out"=w321:errorcluster)  [unwired: 7 in, 1 out]
      }
      frame "WaterInletCloseLDO" {
        n67 = Replace Array Subset(array=w327, new element=FALSE ("new element/subarray"), index=4) -> (w326:bool[])
        n68 = call-poly "Enqueue Message.vi"("error in (no error)"=w330, "Message"="Write bit pattern to FVIR and LDO", "Message Queue"=w334) -> ("error out"=w333:errorcluster)  [unwired: 7 in, 1 out]
      }
      frame "GasSolenoidOpenFVIR" {
        n69 = Replace Array Subset(array=w340, new element=TRUE ("new element/subarray"), index=5) -> (w339:bool[])
        n70 = call-poly "Enqueue Message.vi"("error in (no error)"=w342, "Message"="Write bit pattern to FVIR and LDO", "Message Queue"=w346) -> ("error out"=w345:errorcluster)  [unwired: 7 in, 1 out]
      }
      frame "GasSolenoidOpenLDO" {
        n71 = Replace Array Subset(array=w351, new element=TRUE ("new element/subarray"), index=5) -> (w350:bool[])
        n72 = call-poly "Enqueue Message.vi"("error in (no error)"=w354, "Message"="Write bit pattern to FVIR and LDO", "Message Queue"=w358) -> ("error out"=w357:errorcluster)  [unwired: 7 in, 1 out]
      }
      frame "GasSolenoidCloseFVIR" {
        n73 = Replace Array Subset(array=w364, new element=FALSE ("new element/subarray"), index=5) -> (w363:bool[])
        n74 = call-poly "Enqueue Message.vi"("error in (no error)"=w366, "Message"="Write bit pattern to FVIR and LDO", "Message Queue"=w370) -> ("error out"=w369:errorcluster)  [unwired: 7 in, 1 out]
      }
      frame "GasSolenoidCloseLDO" {
        n75 = Replace Array Subset(array=w375, new element=FALSE ("new element/subarray"), index=5) -> (w374:bool[])
        n76 = call-poly "Enqueue Message.vi"("error in (no error)"=w378, "Message"="Write bit pattern to FVIR and LDO", "Message Queue"=w382) -> ("error out"=w381:errorcluster)  [unwired: 7 in, 1 out]
      }
      frame "WaterFlowOpenFVIR" {
        n77 = Replace Array Subset(array=w388, new element=TRUE ("new element/subarray"), index=6) -> (w387:bool[])
        n78 = call-poly "Enqueue Message.vi"("error in (no error)"=w390, "Message"="Write bit pattern to FVIR and LDO", "Message Queue"=w394) -> ("error out"=w393:errorcluster)  [unwired: 7 in, 1 out]
      }
      frame "WaterFlowStartLDO" {
        n79 = Replace Array Subset(array=w399, new element=TRUE ("new element/subarray"), index=6) -> (w398:bool[])
        n80 = call-poly "Enqueue Message.vi"("error in (no error)"=w402, "Message"="Write bit pattern to FVIR and LDO", "Message Queue"=w406) -> ("error out"=w405:errorcluster)  [unwired: 7 in, 1 out]
      }
      frame "WaterFlowCloseFVIR" {
        n81 = Replace Array Subset(array=w412, new element=FALSE ("new element/subarray"), index=6) -> (w411:bool[])
        n82 = call-poly "Enqueue Message.vi"("error in (no error)"=w414, "Message"="Write bit pattern to FVIR and LDO", "Message Queue"=w418) -> ("error out"=w417:errorcluster)  [unwired: 7 in, 1 out]
      }
      frame "WaterFlowStartZeroLDO" {
        n83 = Replace Array Subset(array=w423, new element=FALSE ("new element/subarray"), index=6) -> (w422:bool[])
        n84 = call-poly "Enqueue Message.vi"("error in (no error)"=w426, "Message"="Write bit pattern to FVIR and LDO", "Message Queue"=w430) -> ("error out"=w429:errorcluster)  [unwired: 7 in, 1 out]
      }
      frame "WaterFlowPropOpenFVIR" {
        n85 = Replace Array Subset(array=w436, new element=TRUE ("new element/subarray"), index=7) -> (w435:bool[])
        n86 = call-poly "Enqueue Message.vi"("error in (no error)"=w438, "Message"="Write bit pattern to FVIR and LDO", "Message Queue"=w442) -> ("error out"=w441:errorcluster)  [unwired: 7 in, 1 out]
      }
      frame "WaterFlowPropOpenLDO" {
        # "This is not used. Remove at some point."
        n87 = Replace Array Subset(array=w447, new element=TRUE ("new element/subarray"), index=7) -> (w446:bool[])
        n88 = call-poly "Enqueue Message.vi"("error in (no error)"=w450, "Message"="Write bit pattern to FVIR and LDO", "Message Queue"=w454) -> ("error out"=w453:errorcluster)  [unwired: 7 in, 1 out]
      }
      frame "WaterFlowPropCloseFVIR" {
        n89 = Replace Array Subset(array=w460, new element=FALSE ("new element/subarray"), index=7) -> (w459:bool[])
        n90 = call-poly "Enqueue Message.vi"("error in (no error)"=w462, "Message"="Write bit pattern to FVIR and LDO", "Message Queue"=w466) -> ("error out"=w465:errorcluster)  [unwired: 7 in, 1 out]
      }
      frame "WaterFlowPropCloseLDO" {
        # "This is not used. Remove at some point."
        n91 = Replace Array Subset(array=w471, new element=FALSE ("new element/subarray"), index=7) -> (w470:bool[])
        n92 = call-poly "Enqueue Message.vi"("error in (no error)"=w474, "Message"="Write bit pattern to FVIR and LDO", "Message Queue"=w478) -> ("error out"=w477:errorcluster)  [unwired: 7 in, 1 out]
      }
      frame "WaterFlowStopLDO" {
        n93 = Replace Array Subset(array=w481, new element=TRUE ("new element/subarray"), index=8) -> (w480:bool[])
        n94 = call-poly "Enqueue Message.vi"("error in (no error)"=w482, "Message"="Write bit pattern to FVIR and LDO", "Message Queue"=w483) -> ("error out"=w479:errorcluster)  [unwired: 7 in, 1 out]
      }
      frame "WaterFlowStopZeroLDO" {
        n95 = Replace Array Subset(array=w495, new element=FALSE ("new element/subarray"), index=8) -> (w494:bool[])
        n96 = call-poly "Enqueue Message.vi"("error in (no error)"=w492, "Message"="Write bit pattern to FVIR and LDO", "Message Queue"=w493) -> ("error out"=w491:errorcluster)  [unwired: 7 in, 1 out]
      }
      frame "OilSpray08Open" {
        n97 = Replace Array Subset(array=w507, new element=TRUE ("new element/subarray"), index=9) -> (w506:bool[])
        n98 = call-poly "Enqueue Message.vi"("error in (no error)"=w510, "Message"="Write bit pattern to FVIR and LDO", "Message Queue"=w514) -> ("error out"=w513:errorcluster)  [unwired: 7 in, 1 out]
      }
      frame "OilSpray08Close" {
        n99 = Replace Array Subset(array=w519, new element=FALSE ("new element/subarray"), index=9) -> (w518:bool[])
        n100 = call-poly "Enqueue Message.vi"("error in (no error)"=w522, "Message"="Write bit pattern to FVIR and LDO", "Message Queue"=w526) -> ("error out"=w525:errorcluster)  [unwired: 7 in, 1 out]
      }
      frame "OilSpray11Open" {
        n101 = Replace Array Subset(array=w531, new element=TRUE ("new element/subarray"), index=10) -> (w530:bool[])
        n102 = call-poly "Enqueue Message.vi"("error in (no error)"=w534, "Message"="Write bit pattern to FVIR and LDO", "Message Queue"=w538) -> ("error out"=w537:errorcluster)  [unwired: 7 in, 1 out]
      }
      frame "OilSpray11Close" {
        n103 = Replace Array Subset(array=w543, new element=FALSE ("new element/subarray"), index=10) -> (w542:bool[])
        n104 = call-poly "Enqueue Message.vi"("error in (no error)"=w546, "Message"="Write bit pattern to FVIR and LDO", "Message Queue"=w550) -> ("error out"=w549:errorcluster)  [unwired: 7 in, 1 out]
      }
      frame "OilSpray133Open" {
        n105 = Replace Array Subset(array=w555, new element=TRUE ("new element/subarray"), index=11) -> (w554:bool[])
        n106 = call-poly "Enqueue Message.vi"("error in (no error)"=w558, "Message"="Write bit pattern to FVIR and LDO", "Message Queue"=w562) -> ("error out"=w561:errorcluster)  [unwired: 7 in, 1 out]
      }
      frame "OilSpray133Close" {
        n107 = Replace Array Subset(array=w567, new element=FALSE ("new element/subarray"), index=11) -> (w566:bool[])
        n108 = call-poly "Enqueue Message.vi"("error in (no error)"=w570, "Message"="Write bit pattern to FVIR and LDO", "Message Queue"=w574) -> ("error out"=w573:errorcluster)  [unwired: 7 in, 1 out]
      }
      frame "HeaterON" {
        n109 = Replace Array Subset(array=w579, new element=FALSE ("new element/subarray"), index=12) -> (w578:bool[])
        n110 = call-poly "Enqueue Message.vi"("error in (no error)"=w582, "Message"="Write bit pattern to FVIR and LDO", "Message Queue"=w586) -> ("error out"=w585:errorcluster)  [unwired: 7 in, 1 out]
      }
      frame "HeaterOFF" {
        n111 = Replace Array Subset(array=w591, new element=TRUE ("new element/subarray"), index=12) -> (w590:bool[])
        n112 = call-poly "Enqueue Message.vi"("error in (no error)"=w594, "Message"="Write bit pattern to FVIR and LDO", "Message Queue"=w598) -> ("error out"=w597:errorcluster)  [unwired: 7 in, 1 out]
      }
      frame "ResetFlowMeter_ON_LDO" {
        n113 = Replace Array Subset(array=w605, new element=TRUE ("new element/subarray"), index=13) -> (w604:bool[])
        n114 = call-poly "Enqueue Message.vi"("error in (no error)"=w601, "Message"="Write bit pattern to FVIR and LDO", "Message Queue"=w602) -> ("error out"=w600:errorcluster)  [unwired: 7 in, 1 out]
      }
      frame "ResetFlowMeter_OFF_LDO" {
        n115 = Replace Array Subset(array=w617, new element=FALSE ("new element/subarray"), index=13) -> (w616:bool[])
        n116 = call-poly "Enqueue Message.vi"("error in (no error)"=w613, "Message"="Write bit pattern to FVIR and LDO", "Message Queue"=w614) -> ("error out"=w612:errorcluster)  [unwired: 7 in, 1 out]
      }
      frame "Water_Heater_Status_ON_LDO" {
        n117 = Replace Array Subset(array=w629, new element=TRUE ("new element/subarray"), index=14) -> (w628:bool[])
        n118 = call-poly "Enqueue Message.vi"("error in (no error)"=w625, "Message"="Write bit pattern to FVIR and LDO", "Message Queue"=w626) -> ("error out"=w624:errorcluster)  [unwired: 7 in, 1 out]
      }
      frame "Water_Heater_Status_OFF_LDO" {
        n119 = Replace Array Subset(array=w641, new element=FALSE ("new element/subarray"), index=14) -> (w640:bool[])
        n120 = call-poly "Enqueue Message.vi"("error in (no error)"=w637, "Message"="Write bit pattern to FVIR and LDO", "Message Queue"=w638) -> ("error out"=w636:errorcluster)  [unwired: 7 in, 1 out]
      }
      frame "PID_Selector_ON" {
        n121 = Replace Array Subset(array=w653, new element=TRUE ("new element/subarray"), index=15) -> (w652:bool[])
        n122 = call-poly "Enqueue Message.vi"("error in (no error)"=w649, "Message"="Write bit pattern to FVIR and LDO", "Message Queue"=w650) -> ("error out"=w648:errorcluster)  [unwired: 7 in, 1 out]
      }
      frame "PID_Selector_OFF" {
        n123 = Replace Array Subset(array=w665, new element=FALSE ("new element/subarray"), index=15) -> (w664:bool[])
        n124 = call-poly "Enqueue Message.vi"("error in (no error)"=w661, "Message"="Write bit pattern to FVIR and LDO", "Message Queue"=w662) -> ("error out"=w660:errorcluster)  [unwired: 7 in, 1 out]
      }
      frame "MannequinGoToHomePos" {
        n125 = Replace Array Subset(array=w680, new element=TRUE ("new element/subarray"), index=9) -> (w679:bool[])
        n126 = call-poly "Enqueue Message.vi"("error in (no error)"=w682, "Message"="Write bit pattern to FVIR and LDO", "Message Queue"=w675) -> ("error out"=w677:errorcluster)  [unwired: 7 in, 1 out]
        n127 = call-poly "Enqueue Message.vi"("error in (no error)"=w677, "Message"="MannequinGoToHomePosClear", "Message Queue"=w675) -> ("error out"=w676:errorcluster)  [unwired: 7 in, 1 out]
      }
      frame "MannequinGoToHomePosClear" {
        n128 = Replace Array Subset(array=w690, new element=FALSE ("new element/subarray"), index=9) -> (w689:bool[])
        n129 = call-poly "Enqueue Message.vi"("error in (no error)"=w692, "Message"="Write bit pattern to FVIR and LDO", "Message Queue"=w696) -> ("error out"=w695:errorcluster)  [unwired: 7 in, 1 out]
      }
      frame "MannequinGoToWorkPos" {
        n130 = Replace Array Subset(array=w706, new element=TRUE ("new element/subarray"), index=10) -> (w705:bool[])
        n131 = call-poly "Enqueue Message.vi"("error in (no error)"=w708, "Message"="Write bit pattern to FVIR and LDO", "Message Queue"=w701) -> ("error out"=w703:errorcluster)  [unwired: 7 in, 1 out]
        n132 = call-poly "Enqueue Message.vi"("error in (no error)"=w703, "Message"="MannequinGoToWorkPosClear", "Message Queue"=w701) -> ("error out"=w702:errorcluster)  [unwired: 7 in, 1 out]
      }
      frame "MannequinGoToWorkPosClear" {
        n133 = Replace Array Subset(array=w716, new element=FALSE ("new element/subarray"), index=10) -> (w715:bool[])
        n134 = call-poly "Enqueue Message.vi"("error in (no error)"=w718, "Message"="Write bit pattern to FVIR and LDO", "Message Queue"=w722) -> ("error out"=w721:errorcluster)  [unwired: 7 in, 1 out]
      }
      frame "SpillCanGoToHomePos" {
        n135 = Replace Array Subset(array=w732, new element=TRUE ("new element/subarray"), index=11) -> (w731:bool[])
        n136 = call-poly "Enqueue Message.vi"("error in (no error)"=w734, "Message"="Write bit pattern to FVIR and LDO", "Message Queue"=w727) -> ("error out"=w729:errorcluster)  [unwired: 7 in, 1 out]
        n137 = call-poly "Enqueue Message.vi"("error in (no error)"=w729, "Message"="SpillCanGoToHomePosClear", "Message Queue"=w727) -> ("error out"=w728:errorcluster)  [unwired: 7 in, 1 out]
      }
      frame "SpillCanGoToHomePosClear" {
        n138 = Replace Array Subset(array=w742, new element=FALSE ("new element/subarray"), index=11) -> (w741:bool[])
        n139 = call-poly "Enqueue Message.vi"("error in (no error)"=w744, "Message"="Write bit pattern to FVIR and LDO", "Message Queue"=w748) -> ("error out"=w747:errorcluster)  [unwired: 7 in, 1 out]
      }
      frame "SpillCanGoToWorkPos" {
        n140 = Replace Array Subset(array=w758, new element=TRUE ("new element/subarray"), index=12) -> (w757:bool[])
        n141 = call-poly "Enqueue Message.vi"("error in (no error)"=w760, "Message"="Write bit pattern to FVIR and LDO", "Message Queue"=w753) -> ("error out"=w755:errorcluster)  [unwired: 7 in, 1 out]
        n142 = call-poly "Enqueue Message.vi"("error in (no error)"=w755, "Message"="SpillCanGoToWorkPosClear", "Message Queue"=w753) -> ("error out"=w754:errorcluster)  [unwired: 7 in, 1 out]
      }
      frame "SpillCanGoToWorkPosClear" {
        n143 = Replace Array Subset(array=w768, new element=FALSE ("new element/subarray"), index=12) -> (w767:bool[])
        n144 = call-poly "Enqueue Message.vi"("error in (no error)"=w770, "Message"="Write bit pattern to FVIR and LDO", "Message Queue"=w774) -> ("error out"=w773:errorcluster)  [unwired: 7 in, 1 out]
      }
      frame "TestCase1Winter" {
        # "Writing to PLC with value 1 at address 7"
        n145 = call-dynamic "Write Single Holding Register.vi"("error in"=w787, "register to write"=u16 1, "address"=u16 7 ("starting address"), "Modbus master in"=w785) -> ("error out"=w781:errorcluster, "Modbus master out"=w786:refnum<class "Modbus Master.lvclass">)  [unwired: 6 in]
        n146 = call-poly "Enqueue Message.vi"("error in (no error)"=w781, "Message"="Write bit pattern to FVIR and LDO", "Message Queue"=w782) -> ("error out"=w779:errorcluster)  [unwired: 7 in, 1 out]
      }
      frame "TestCase1Summer" {
        # "Writing to PLC with value 2 at address 7"
        n147 = call-dynamic "Write Single Holding Register.vi"("error in"=w800, "register to write"=u16 2, "address"=u16 7 ("starting address"), "Modbus master in"=w798) -> ("error out"=w794:errorcluster, "Modbus master out"=w799:refnum<class "Modbus Master.lvclass">)  [unwired: 6 in]
        n148 = call-poly "Enqueue Message.vi"("error in (no error)"=w794, "Message"="Write bit pattern to FVIR and LDO", "Message Queue"=w795) -> ("error out"=w792:errorcluster)  [unwired: 7 in, 1 out]
      }
      frame "TestCase2Winter" {
        # "Writing to PLC with value 3 at address 7"
        n149 = call-dynamic "Write Single Holding Register.vi"("error in"=w813, "register to write"=u16 3, "address"=u16 7 ("starting address"), "Modbus master in"=w811) -> ("error out"=w807:errorcluster, "Modbus master out"=w812:refnum<class "Modbus Master.lvclass">)  [unwired: 6 in]
        n150 = call-poly "Enqueue Message.vi"("error in (no error)"=w807, "Message"="Write bit pattern to FVIR and LDO", "Message Queue"=w808) -> ("error out"=w805:errorcluster)  [unwired: 7 in, 1 out]
      }
      frame "TestCase2Summer" {
        # "Writing to PLC with value 4 at address 7"
        n151 = call-dynamic "Write Single Holding Register.vi"("error in"=w826, "register to write"=u16 4, "address"=u16 7 ("starting address"), "Modbus master in"=w824) -> ("error out"=w820:errorcluster, "Modbus master out"=w825:refnum<class "Modbus Master.lvclass">)  [unwired: 6 in]
        n152 = call-poly "Enqueue Message.vi"("error in (no error)"=w820, "Message"="Write bit pattern to FVIR and LDO", "Message Queue"=w821) -> ("error out"=w818:errorcluster)  [unwired: 7 in, 1 out]
      }
      frame "TestCase3Winter" {
        # "Writing to PLC with value 5 at address 7"
        n153 = call-dynamic "Write Single Holding Register.vi"("error in"=w839, "register to write"=u16 5, "address"=u16 7 ("starting address"), "Modbus master in"=w837) -> ("error out"=w833:errorcluster, "Modbus master out"=w838:refnum<class "Modbus Master.lvclass">)  [unwired: 6 in]
        n154 = call-poly "Enqueue Message.vi"("error in (no error)"=w833, "Message"="Write bit pattern to FVIR and LDO", "Message Queue"=w834) -> ("error out"=w831:errorcluster)  [unwired: 7 in, 1 out]
      }
      frame "TestCase3Summer" {
        # "Writing to PLC with value 6 at address 7"
        n155 = call-dynamic "Write Single Holding Register.vi"("error in"=w852, "register to write"=u16 6, "address"=u16 7 ("starting address"), "Modbus master in"=w850) -> ("error out"=w846:errorcluster, "Modbus master out"=w851:refnum<class "Modbus Master.lvclass">)  [unwired: 6 in]
        n156 = call-poly "Enqueue Message.vi"("error in (no error)"=w846, "Message"="Write bit pattern to FVIR and LDO", "Message Queue"=w847) -> ("error out"=w844:errorcluster)  [unwired: 7 in, 1 out]
      }
      frame "TestCase4Winter" {
        # "Writing to PLC with value 7 at address 7"
        n157 = call-dynamic "Write Single Holding Register.vi"("error in"=w857, "register to write"=u16 7, "address"=u16 7 ("starting address"), "Modbus master in"=w864) -> ("error out"=w860:errorcluster, "Modbus master out"=w865:refnum<class "Modbus Master.lvclass">)  [unwired: 6 in]
        n158 = call-poly "Enqueue Message.vi"("error in (no error)"=w860, "Message"="Write bit pattern to FVIR and LDO", "Message Queue"=w861) -> ("error out"=w858:errorcluster)  [unwired: 7 in, 1 out]
      }
      frame "TestCase4Summer" {
        # "Writing to PLC with value 8 at address 7"
        n159 = call-dynamic "Write Single Holding Register.vi"("error in"=w878, "register to write"=u16 8, "address"=u16 7 ("starting address"), "Modbus master in"=w876) -> ("error out"=w872:errorcluster, "Modbus master out"=w877:refnum<class "Modbus Master.lvclass">)  [unwired: 6 in]
        n160 = call-poly "Enqueue Message.vi"("error in (no error)"=w872, "Message"="Write bit pattern to FVIR and LDO", "Message Queue"=w873) -> ("error out"=w870:errorcluster)  [unwired: 7 in, 1 out]
      }
      frame "ResetTestFVIR" {
        # "Writing to PLC with value 0 at address 7"
        n161 = call-dynamic "Write Single Holding Register.vi"("error in"=w891, "register to write"=u16 0, "address"=u16 7 ("starting address"), "Modbus master in"=w889) -> ("error out"=w885:errorcluster, "Modbus master out"=w890:refnum<class "Modbus Master.lvclass">)  [unwired: 6 in]
        n162 = call-poly "Enqueue Message.vi"("error in (no error)"=w885, "Message"="Write bit pattern to FVIR and LDO", "Message Queue"=w886) -> ("error out"=w883:errorcluster)  [unwired: 7 in, 1 out]
      }
      frame "ResetTestLDO" {
        # "Writing to PLC with value 0 at address 10"
        n163 = call-dynamic "Write Single Holding Register.vi"("error in"=w904, "register to write"=u16 0, "address"=u16 10 ("starting address"), "Modbus master in"=w902) -> ("error out"=w898:errorcluster, "Modbus master out"=w903:refnum<class "Modbus Master.lvclass">)  [unwired: 6 in]
        n164 = call-poly "Enqueue Message.vi"("error in (no error)"=w898, "Message"="Write bit pattern to FVIR and LDO", "Message Queue"=w899) -> ("error out"=w896:errorcluster)  [unwired: 7 in, 1 out]
      }
      frame "SendParamToPLCFVIR" {
        # "This for loop basically just takes the array from the Modbus queue and write\neach index value to each unique register. I.e. the first control value from the HMI\nwhich is \"Time delay of change direction of mannequin actuators\" is written to \nregister 1 (40002). The next control value from the HMI is the \"Number of\nmannequin movement\" and that value is written to register 2 (40003). \nThis continues until there are no further values in the array.\n\n(Register 0 is the bit combination from, regsiter 40001). See\nthe case  \"Writing to register 40001)"
        n165 = Variant To Data(type=i32[] [], Variant=w917) -> (data=w913:i32[], error out=w910:errorcluster)  [unwired: 1 in]
        n166 = Array Size(array=w913) -> (size(s)=w914:i32)
        n167 = for {
          N: w914 -> [_]
          tunnel: w913 -> [w928]
          shift-right: [w922] -> w911
          shift-left: w912 -> [w923]
          shift-right: [w920] -> w909
          shift-left: w910 -> [w921]
          i -> [w926]
          n168 = Index Array(array=w928, index=w926) -> (element=w927:i32)
          n169 = Add(x=1, y=w926) -> (x+y=w924:i32)
          n170 = call-dynamic "Write Single Holding Register.vi"("error in"=w921, "register to write"=w927, "address"=w924, "Modbus master in"=w923) -> ("error out"=w920:errorcluster, "Modbus master out"=w922:refnum<class "Modbus Master.lvclass">)  [unwired: 6 in]
        }
        n171 = call-poly "Enqueue Message.vi"("error in (no error)"=w909, "Message"="Write bit pattern to FVIR and LDO", "Message Queue"=w919) -> ("error out"=w915:errorcluster)  [unwired: 7 in, 1 out]
      }
      frame "SendParamToPLCLDO" {
        # "This for loop basically just takes the array from the Modbus queue and write\neach index value to each unique register. I.e. the first control value from the HMI\nwhich is \"Time delay of change direction of mannequin actuators\" is written to \nregister 1 (40002). The next control value from the HMI is the \"Number of\nmannequin movement\" and that value is written to register 2 (40003). \nThis continues until there are no further values in the array.\n\n(Register 0 is the bit combination from, regsiter 40001). See\nthe case  \"Writing to register 40001)"
        n172 = Variant To Data(type=i32[] [], Variant=w940) -> (data=w937:i32[], error out=w934:errorcluster)  [unwired: 1 in]
        n173 = call "Modbus Send Parameters LDO.vi"("error in (no error)"=w934, "Array in"=w937, "Modbus Master in"=w936) -> ("error out"=w933:errorcluster, "Modbus Master out"=w935:refnum<class "Modbus Master.lvclass">)  [unwired: 7 in]
        n174 = call-poly "Enqueue Message.vi"("error in (no error)"=w933, "Message"="Write bit pattern to FVIR and LDO", "Message Queue"=w942) -> ("error out"=w938:errorcluster)  [unwired: 7 in, 1 out]
      }
      frame "Reset all button signals to PLC" {
        # "Reset all the buttons signals after watchdog pause."
        n175 = call-dynamic "Write Multiple Holding Registers.vi"("error in"=w952, "registers to write"=u16[] [99, 99, 99, 99, 99, 99, 99, 99, 99, 99, 99, 99], "starting address"=u16 10, "Modbus master in"=w950) -> ("error out"=w948:errorcluster, "Modbus master out"=w951:refnum<class "Modbus Master.lvclass">)  [unwired: 6 in]
      }
      frame "Disconnect" {
        # "I moved this to the Exit State. Would like to eliminate the \"Connect\" and \"Disconnect\" button"
        # "Flushing the WD helper loop in order to quick close down, if the operator is pressing Exit"
        n176 = call-dynamic "Shutdown.vi"("error in"=w963, "Modbus master in"=w962) -> ("error out"=w964:errorcluster)  [unwired: 9 in]
        n177 = call <vilib>:"Clear Errors.vi"("error in (no error)"=w964) -> ("error out"=w961:errorcluster)  [unwired: 5 in, 1 out]
        n178 = Flush Queue(queue=w960, error in (no error)=w961) -> (error out=w957:errorcluster)  [unwired: 2 out]
        n179 = case shown="No Error" w957 {
          selector: w957 -> [w973 w976]
          tunnel: w955 -> [w965 w974]
          tunnel: [w971 w975] -> w956
          frame No Error {
            n180 = call-poly "Enqueue Message.vi"("error in (no error)"=w973, "Message Data"="Succesfully disconnected with Modbus TCP/IP..." ("Acquiring and Logging..."), "Message"="Update Status - FVIR", "Message Queue"=w965) -> ("error out"=w972:errorcluster, "dup Message Queue"=w970:refnum<queue>)  [unwired: 6 in]
            n181 = call-poly "Enqueue Message.vi"("error in (no error)"=w972, "Message Data"="Succesfully disconnected with Modbus TCP/IP..." ("Acquiring and Logging..."), "Message"="Update Status - LDO", "Message Queue"=w970) -> ("error out"=w971:errorcluster)  [unwired: 6 in, 1 out]
          }
          frame Error {
            n182 = call-poly "Enqueue Message.vi"("error in (no error)"=w976, "Message Data"="Error with disconnecting with Modbus TCP/IP..." ("Acquiring and Logging..."), "Message"="Update Status - FVIR", "Message Queue"=w974) -> ("error out"=w982:errorcluster, "dup Message Queue"=w981:refnum<queue>)  [unwired: 6 in]
            n183 = call-poly "Enqueue Message.vi"("error in (no error)"=w982, "Message Data"="Error with disconnecting with Modbus TCP/IP..." ("Acquiring and Logging..."), "Message"="Update Status - LDO", "Message Queue"=w981) -> ("error out"=w975:errorcluster)  [unwired: 6 in, 1 out]
          }
        }
      }
      frame "Exit" {
        # "Flushing the WD helper loop in order to quick close down, if the operator is pressing Exit"
        # "When main loop receive \"Exit\" on its queue, the exit case will commit \"Exit\" to its helper loop"
        # "Stop the VI"
        n184 = Flush Queue(queue=w990, error in (no error)=w991) -> (queue out=w989:refnum<queue>, error out=w988:errorcluster)  [unwired: 1 out]
        n185 = call-dynamic "Shutdown.vi"("error in"=w988, "Modbus master in"=w987) -> ("error out"=w992:errorcluster)  [unwired: 9 in]
        n186 = call <vilib>:"Clear Errors.vi"("error in (no error)"=w992) -> ("error out"=w986:errorcluster)  [unwired: 5 in, 1 out]
        n187 = case shown="No Error" w986 {
          selector: w986 -> [w1010 w1013]
          tunnel: w983 -> [w1002 w1011]
          tunnel: [w1008 w1012] -> w985
          frame No Error {
            n188 = call-poly "Enqueue Message.vi"("error in (no error)"=w1010, "Message Data"="Succesfully disconnected with Modbus TCP/IP..." ("Acquiring and Logging..."), "Message"="Update Status - FVIR", "Message Queue"=w1002) -> ("error out"=w1009:errorcluster, "dup Message Queue"=w1007:refnum<queue>)  [unwired: 6 in]
            n189 = call-poly "Enqueue Message.vi"("error in (no error)"=w1009, "Message Data"="Succesfully disconnected with Modbus TCP/IP..." ("Acquiring and Logging..."), "Message"="Update Status - LDO", "Message Queue"=w1007) -> ("error out"=w1008:errorcluster)  [unwired: 6 in, 1 out]
          }
          frame Error {
            n190 = call-poly "Enqueue Message.vi"("error in (no error)"=w1013, "Message Data"="Error with disconnecting with Modbus TCP/IP..." ("Acquiring and Logging..."), "Message"="Update Status - FVIR", "Message Queue"=w1011) -> ("error out"=w1019:errorcluster, "dup Message Queue"=w1018:refnum<queue>)  [unwired: 6 in]
            n191 = call-poly "Enqueue Message.vi"("error in (no error)"=w1019, "Message Data"="Error with disconnecting with Modbus TCP/IP..." ("Acquiring and Logging..."), "Message"="Update Status - LDO", "Message Queue"=w1018) -> ("error out"=w1012:errorcluster)  [unwired: 6 in, 1 out]
          }
        }
        n192 = call-poly "Enqueue Message.vi"("Priority Message? (F)"=TRUE, "error in (no error)"=w985, "Message"="Exit", "Message Queue"=w989) -> ("error out"=w997:errorcluster)  [unwired: 6 in, 1 out]
        n193 = Release Queue(queue=w1001, error in (no error)=w997) -> (error out=w984:errorcluster)  [unwired: 1 in, 2 out]
      }
      frame "ValveChangeEPV" {
        n194 = Variant To Data(error in=w1032, type=0.0 ("Numeric"), Variant=w1031) -> (data=w1029:dbl, error out=w1030:errorcluster)
        n195 = call "UTILITY Modbus 32bit Number to 16bit Array.vi"("error in"=w1030, "32-bit IEEE 754"=w1029) -> ("error out"=w1028:errorcluster, "U16 Array Representation"=w1026:u16[])  [unwired: 8 in]
        n196 = call-dynamic "Write Multiple Holding Registers.vi"("error in"=w1028, "registers to write"=w1026, "starting address"=u16 11 ("address"), "Modbus master in"=w1025) -> ("error out"=w1022:errorcluster, "Modbus master out"=w1024:refnum<class "Modbus Master.lvclass">)  [unwired: 6 in]
        n197 = call-poly "Enqueue Message.vi"("error in (no error)"=w1022, "Message"="Write bit pattern to FVIR and LDO", "Message Queue"=w1020) -> ("error out"=w1021:errorcluster)  [unwired: 7 in, 1 out]
      }
      frame "TempChangeDRK375" {
        n198 = Variant To Data(error in=w1050, type=0.0 ("Numeric"), Variant=w1049) -> (data=w1044:dbl, error out=w1045:errorcluster)
        n199 = call "UTILITY Modbus 32bit Number to 16bit Array.vi"("error in"=w1045, "32-bit IEEE 754"=w1044) -> ("error out"=w1048:errorcluster, "U16 Array Representation"=w1046:u16[])  [unwired: 8 in]
        n200 = call-dynamic "Write Multiple Holding Registers.vi"("error in"=w1048, "registers to write"=w1046, "starting address"=u16 13 ("address"), "Modbus master in"=w1043) -> ("error out"=w1039:errorcluster, "Modbus master out"=w1042:refnum<class "Modbus Master.lvclass">)  [unwired: 6 in]
        n201 = call-poly "Enqueue Message.vi"("error in (no error)"=w1039, "Message"="Write bit pattern to FVIR and LDO", "Message Queue"=w1040) -> ("error out"=w1038:errorcluster)  [unwired: 7 in, 1 out]
      }
      frame "ValveChangeDRK375" {
        n202 = Variant To Data(error in=w1068, type=0.0 ("Numeric"), Variant=w1067) -> (data=w1062:dbl, error out=w1063:errorcluster)
        n203 = call "UTILITY Modbus 32bit Number to 16bit Array.vi"("error in"=w1063, "32-bit IEEE 754"=w1062) -> ("error out"=w1066:errorcluster, "U16 Array Representation"=w1065:u16[])  [unwired: 8 in]
        n204 = call-dynamic "Write Multiple Holding Registers.vi"("error in"=w1066, "registers to write"=w1065, "starting address"=u16 15 ("address"), "Modbus master in"=w1061) -> ("error out"=w1057:errorcluster, "Modbus master out"=w1060:refnum<class "Modbus Master.lvclass">)  [unwired: 6 in]
        n205 = call-poly "Enqueue Message.vi"("error in (no error)"=w1057, "Message"="Write bit pattern to FVIR and LDO", "Message Queue"=w1058) -> ("error out"=w1056:errorcluster)  [unwired: 7 in, 1 out]
      }
      frame "Output_Temperature_Target" {
        n206 = Variant To Data(error in=w1081, type=0.0 ("Numeric"), Variant=w1080) -> (data=w1084:dbl, error out=w1085:errorcluster)
        n207 = call "UTILITY Modbus 32bit Number to 16bit Array.vi"("error in"=w1085, "32-bit IEEE 754"=w1084) -> ("error out"=w1087:errorcluster, "U16 Array Representation"=w1086:u16[])  [unwired: 8 in]
        n208 = call-dynamic "Write Multiple Holding Registers.vi"("error in"=w1087, "registers to write"=w1086, "starting address"=u16 17 ("address"), "Modbus master in"=w1079) -> ("error out"=w1076:errorcluster, "Modbus master out"=w1078:refnum<class "Modbus Master.lvclass">)  [unwired: 6 in]
        n209 = call-poly "Enqueue Message.vi"("error in (no error)"=w1076, "Message"="Write bit pattern to FVIR and LDO", "Message Queue"=w1074) -> ("error out"=w1075:errorcluster)  [unwired: 7 in, 1 out]
      }
      frame "Output_Flow_Target" {
        n210 = Variant To Data(error in=w1099, type=0.0 ("Numeric"), Variant=w1098) -> (data=w1102:dbl, error out=w1103:errorcluster)
        n211 = call "UTILITY Modbus 32bit Number to 16bit Array.vi"("error in"=w1103, "32-bit IEEE 754"=w1102) -> ("error out"=w1105:errorcluster, "U16 Array Representation"=w1104:u16[])  [unwired: 8 in]
        n212 = call-dynamic "Write Multiple Holding Registers.vi"("error in"=w1105, "registers to write"=w1104, "starting address"=u16 31 ("address"), "Modbus master in"=w1097) -> ("error out"=w1094:errorcluster, "Modbus master out"=w1096:refnum<class "Modbus Master.lvclass">)  [unwired: 6 in]
        n213 = call-poly "Enqueue Message.vi"("error in (no error)"=w1094, "Message"="Write bit pattern to FVIR and LDO", "Message Queue"=w1092) -> ("error out"=w1093:errorcluster)  [unwired: 7 in, 1 out]
      }
    }
    n214 = Build Array (concatenate)(w9, w8) -> (w7:string[])
    "appended array" <- w7
    n215 = call "Error Handler - Message Handling Loop.vi"("error in (no error)"=w19, "Message Queue"=w27) -> ("dup error in"=w31:errorcluster)  [unwired: 8 in, 1 out]
    "Loop Count" <- w10
  }
  n216 = Merge Errors(w3) -> (→"error out":errorcluster)
